vi "Check_Execution_Row.vi"(0 "Execution Row":T1 {"Carrier_2 Q (l/min)" format="%#.2f"; "Row Duration (mins)" format="%#.1f"; "Row No" min=0; "Trace Gas Concentration (%)" min=0.0 format="%#_4f"; "Carrier_1 Q (l/min)" format="%#.2f"; "Tunnel Speed" format="%#.2f"; "Start X" format="%#.2f"; "Start Y" format="%#.2f"; "Start Z" format="%#.2f"; "End X" format="%#.2f"; "End Y" format="%#.2f"; "End Z" format="%#.2f"; "Averaging time (min)" min=0.0 format="%#.2f"}, 1 "Earlier Filenames":path[](array[path]), 3 "Synchronization Start No":i32=1 min=1 max=100, 4 "Row Index":i32, 5 "Max Tunnel Speed":dbl format="%.2f") -> (6 "Edited Row":bool, 7 "Execution Row Out":T1 {"Carrier_2 Q (l/min)" format="%#.2f"; "Row Duration (mins)" format="%#.1f"; "Row No" min=0; "Trace Gas Concentration (%)" min=0.0 format="%#_4f"; "Carrier_1 Q (l/min)" format="%#.2f"; "Tunnel Speed" format="%#.2f"; "Start X" format="%#.2f"; "Start Y" format="%#.2f"; "Start Z" format="%#.2f"; "End X" format="%#.2f"; "End Y" format="%#.2f"; "End Z" format="%#.2f"; "Averaging time (min)" min=0.0 format="%#.2f"}, 9 "Continue?":bool, 10 "Error Comments":string)   [LabVIEW 2016]
uses:
  Traverse_cluster.ctl
  Spacing.ctl
  Controls/Multi_run_mode.ctl
  Controls/User_Specific_mode.ctl
  Controls/Home.ctl
  Controls/Tunnel_Coordinates.ctl
  ADAM Client/Sub VIs/ADAM Controls/Channel_names.ctl
  Globals/Extra_Commands_Global.vi
  Globals/Constants_global.vi
  Globals/Trav_pos_global.vi
panel:
  out "Traverse line Out":T1 {"Carrier_2 Q (l/min)" format="%#.2f"; "Row Duration (mins)" format="%#.1f"; "Row No" min=0; "Trace Gas Concentration (%)" min=0.0 format="%#_4f"; "Carrier_1 Q (l/min)" format="%#.2f"; "Tunnel Speed" format="%#.2f"; "Start X" format="%#.2f"; "Start Y" format="%#.2f"; "Start Z" format="%#.2f"; "End X" format="%#.2f"; "End Y" format="%#.2f"; "End Z" format="%#.2f"; "Averaging time (min)" min=0.0 format="%#.2f"}
  out "Fixed Axis":bool[](array[boolean])
  out "Filenames":string[](array[string])
  out "Current Sync Number":i32
  out "Checks":string[](array[string])
  in  "Edit in Excel":bool
  in  "OK":bool
  # "X           Y            Z"
  # "Start"
  # "End"
  # "X           Y            Z"
  # "Start"
  # "End"
  # "X           Y            Z"
  # "Start"
  # "End"
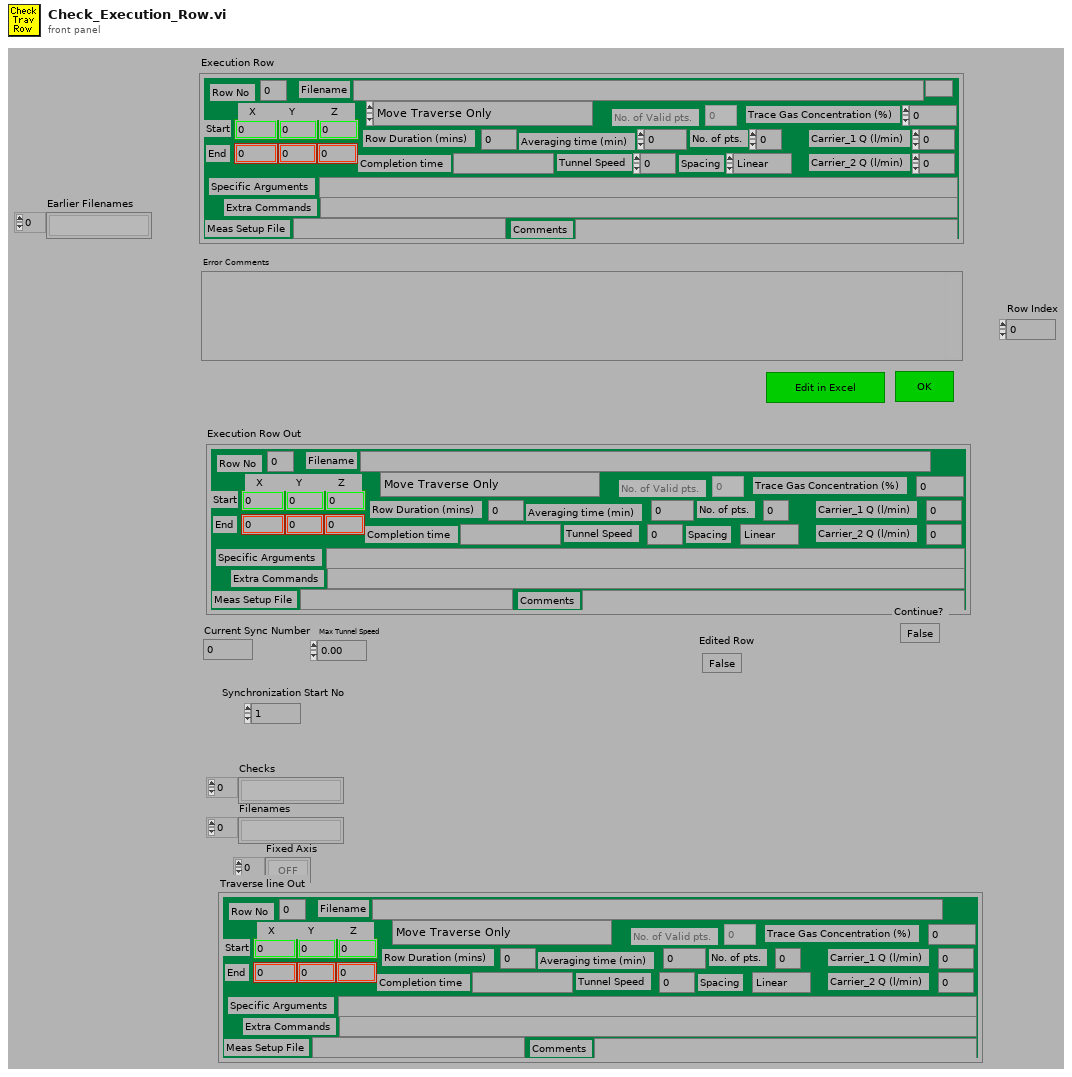
[diagram p1: front panel]
types:
  T1 = typedef "Traverse_cluster.ctl" = cluster{"Start X":sgl, "Start Y":sgl, "Start Z":sgl, "End X":sgl, "End Y":sgl, "End Z":sgl, "No. of pts.":i32, "Spacing":T2, "Filename":path, "Tunnel Speed":dbl, "Averaging time (min)":dbl, "Extra Commands":string, "Carrier_1 Q (l/min)":dbl, "Carrier_2 Q (l/min)":dbl, "Trace Gas Concentration (%)":dbl, "Specific Arguments":string, "Comments":string, "Row No":i32, "Row Type Selector":T3, "Completion time":string, "Row Duration (mins)":dbl, "No. of Valid pts.":i32, "Meas Setup File":string}
  T2 = typedef "Spacing.ctl" = enum16{"Linear", "Log", "Gauss", "Specified", "N/A"}
  T3 = typedef "Multi_run_mode.ctl" = enum16{"Move Traverse Only", "Set Tunnel Speed Only", "Set Source Only", "Set Measurement Conditions", "Single Measurement", "Vertical Profile", "Lateral Profile", "Longitudinal Profile", "Explore Volume", "Multi-Axis Profile", "Auto Calibrate", "Meas Fast FID Bkgnd", "Check Beam Power", "Scanning Valve Measurement", "Run VI Named:", "Set ADAM Ch", "Wait (minutes)", "Send Message", "Synchronize With:", "Fall Back to this Row", "Turn Off Row Repeating", "Blank Row", "Traverse 3D Volume"}
  T4 = enum16{"All Channel Names", "Valid Channel Names"}
  T5 = typedef "User_Specific_mode.ctl" = enum16{"Check VI only", "Run VI"}
  T6 = typedef "Home.ctl" = enum16{"Don't Home", "Home  +X", "Home  -X", "Home  +Y", "Home  -Y", "Home  +Z", "Home  -Z"}
  T7 = typedef "Tunnel_Coordinates.ctl" = enum16{"Work in Tunnel Coordinates", "Work in Model Coordinates"}
  T8 = enum16{"Zero or one", "One", "Zero or more", "One or more"}
  T9 = typedef "Channel_names.ctl" = enum16{"Active Only", "Active + Off", "All Channels"}
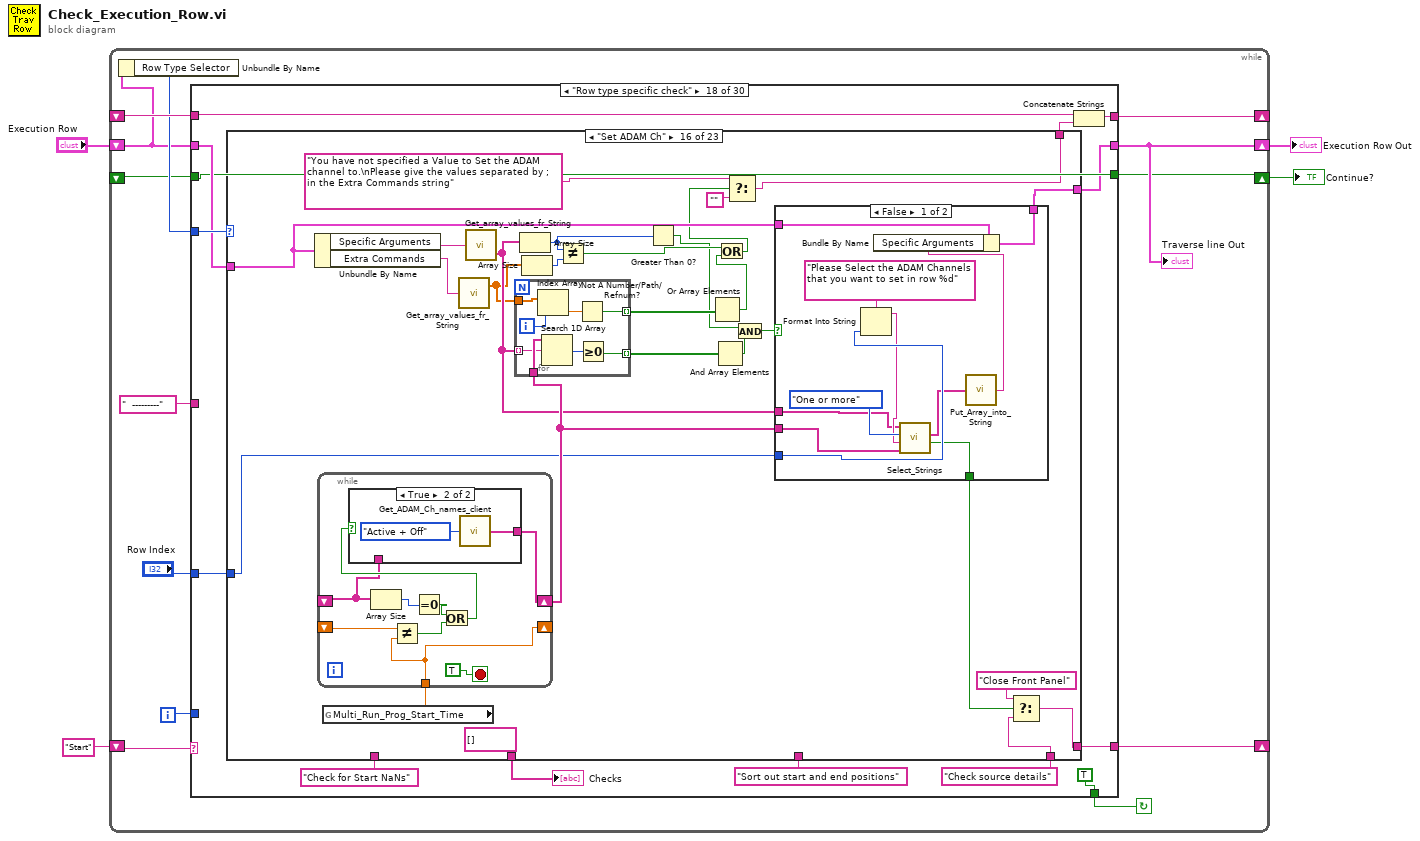
[diagram p0: block diagram]
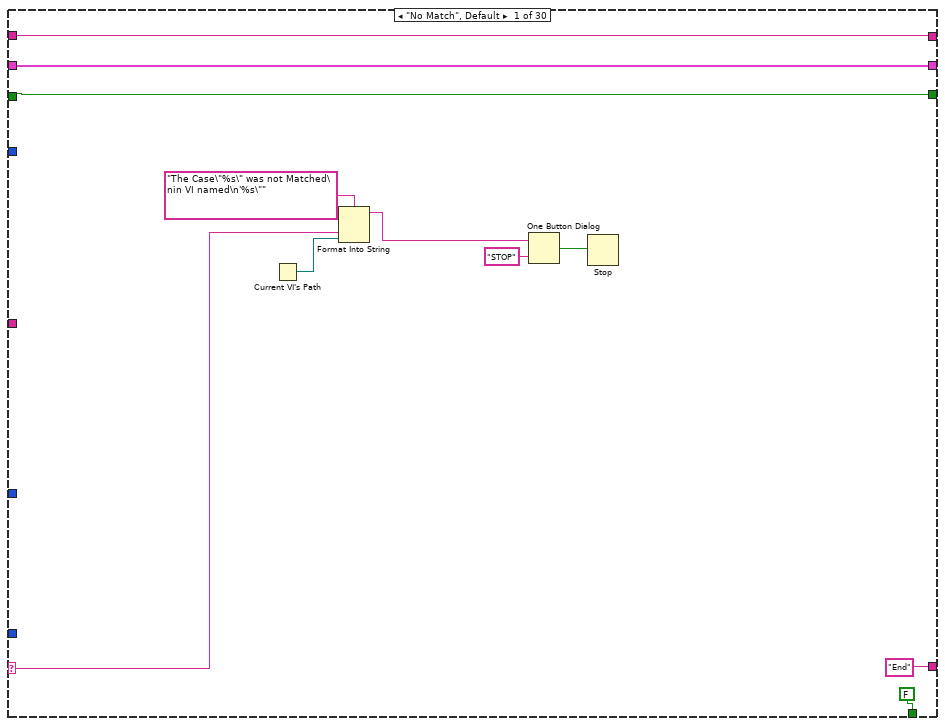
[diagram p2: hidden frame]
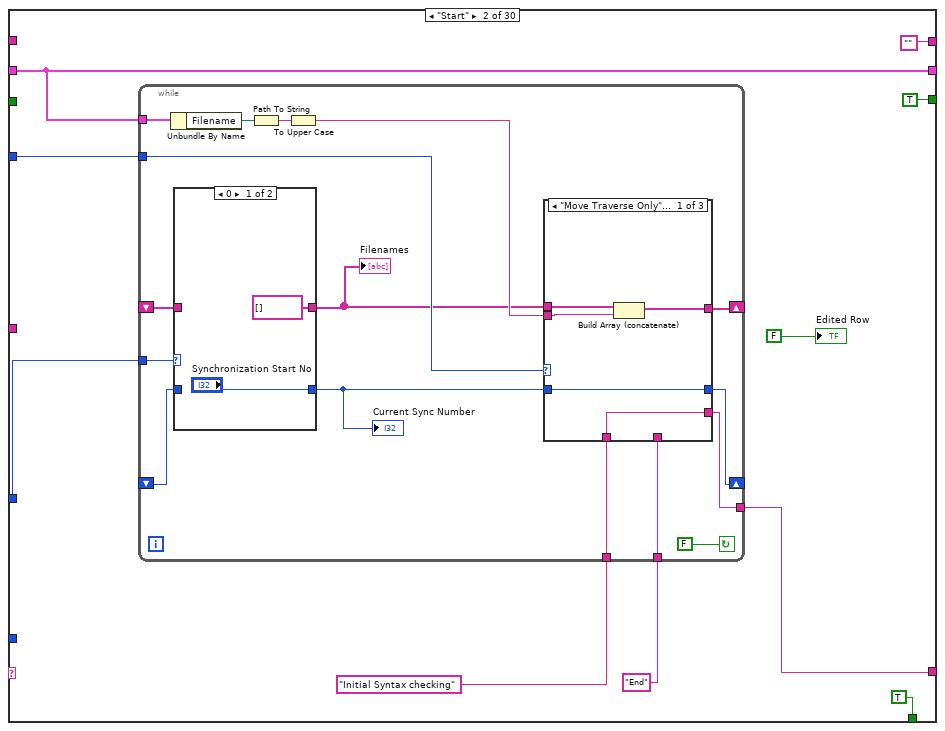
[diagram p3: hidden frame]
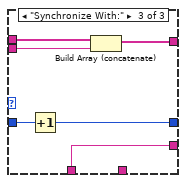
[diagram p6: hidden frame]
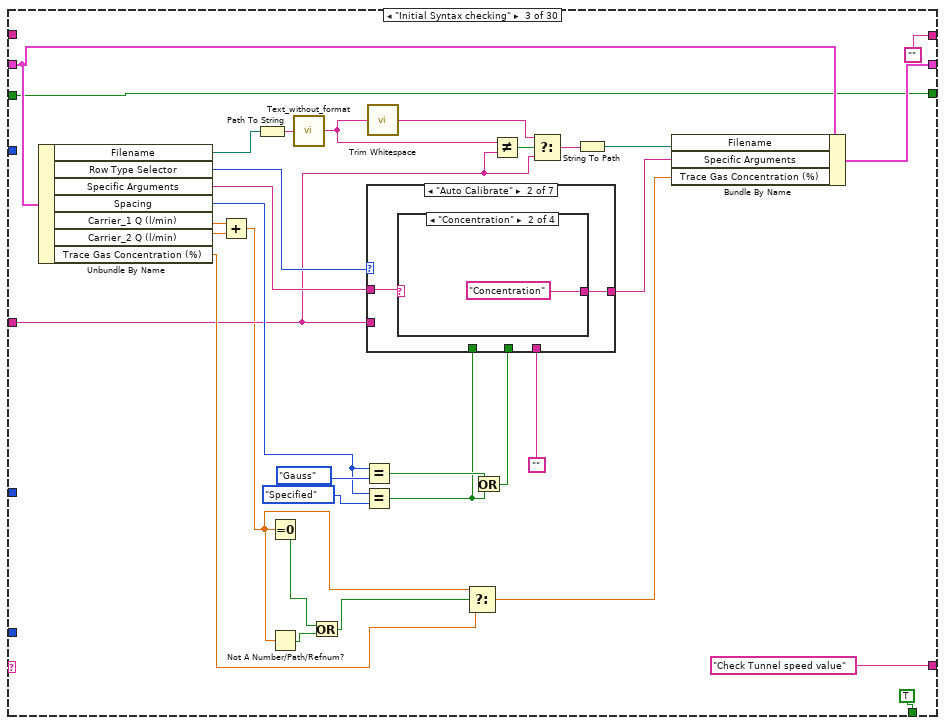
[diagram p7: hidden frame]
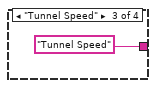
[diagram p10: hidden frame]
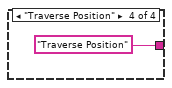
[diagram p11: hidden frame]
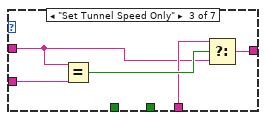
[diagram p12: hidden frame]
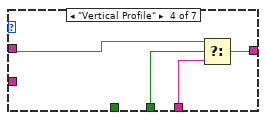
[diagram p13: hidden frame]
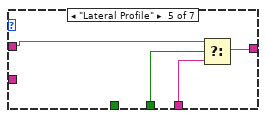
[diagram p14: hidden frame]
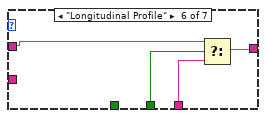
[diagram p15: hidden frame]
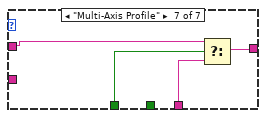
[diagram p16: hidden frame]
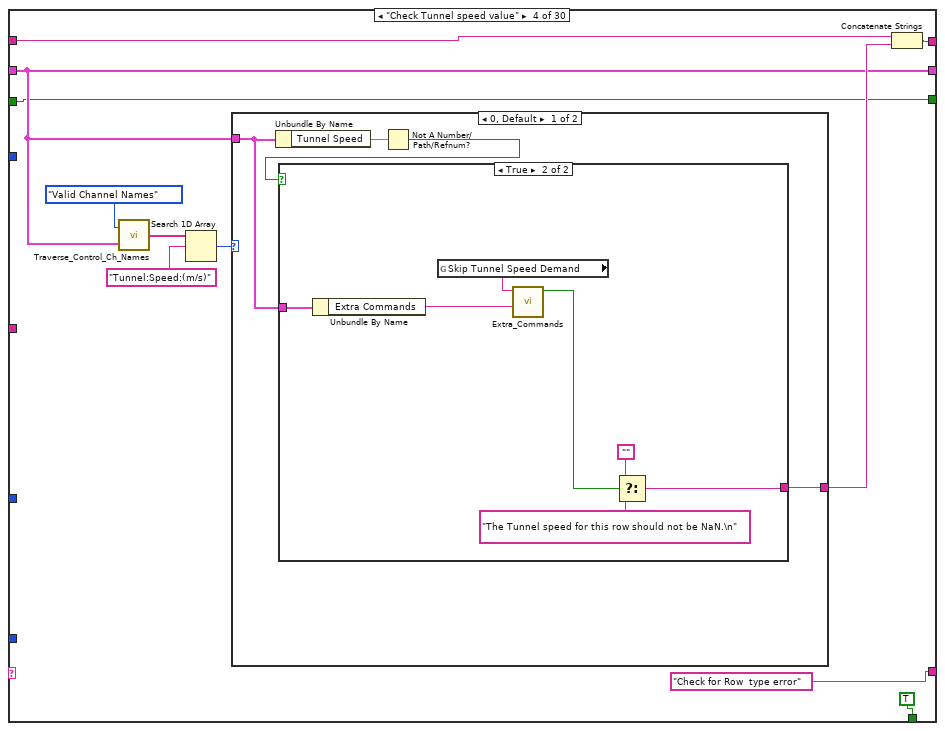
[diagram p17: hidden frame]
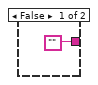
[diagram p18: hidden frame]
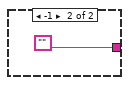
[diagram p19: hidden frame]
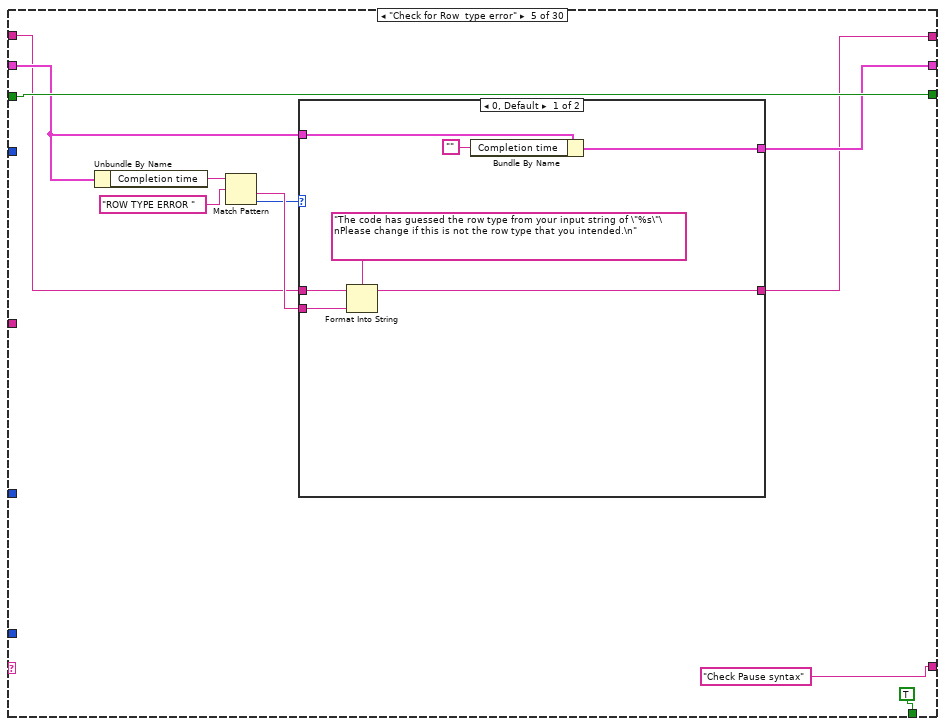
[diagram p20: hidden frame]
diagram:
  n1 = while {
    shift-left: _ -> [w16]
    shift-right: [w17] -> _
    shift-left: "Start" -> [w9]
    shift-right: [w14] -> _
    shift-right: [w8] -> w2
    shift-left: "Execution Row" -> [w5]
    shift-right: [w7] -> w1
    shift-left: _ -> [w6]
    i -> [w10]
    stop <- w15 continue-if-true
    n2 = Unbundle By Name(w5) -> ("Row Type Selector"=w12:T3)
    n3 = case shown="\"Row type specific check\"" w9 {
      tunnel: w5 -> [w23 w32 w99 w136 w160 w192 w217 w264 w294 w324 w357 w433 w460 w499 w555 w587 w595 w634 w1005 w1105 w1142 w1173 w1255 w1266 w1274 w1342 _ w1379 w1386 w1396]
      tunnel: "  ---------" ("f") -> [_ _ w77 _ _ w196 _ _ _ _ _ _ _ _ _ _ _ _ _ _ _ _ _ _ _ _ _ _ _ _]
      tunnel: "Row Index" -> [_ w36 _ _ _ _ w214 _ _ _ _ _ _ _ _ _ _ w628 _ _ _ _ _ _ _ _ _ w1380 _ w1395]
      selector: w9 -> [w18 _ _ _ _ _ _ _ _ _ _ _ _ _ _ _ _ _ _ _ _ _ _ _ _ _ _ _ _ _]
      tunnel: [w22 "" "" w137 w157 w185 w223 w265 w295 w325 w359 w437 w463 w504 w557 w591 w600 w638 w1010 w1115 w1148 w1196 w1254 w1268 w1275 w1348 w1357 w1381 w1391 w1398] -> w17
      tunnel: w12 -> [_ w35 _ _ _ w178 _ _ _ _ _ _ _ _ _ _ w598 w637 w1006 w1103 _ _ _ _ w1279 _ _ _ _ _]
      tunnel: w16 -> [w22 _ _ w138 w158 w187 w224 w266 w296 w326 w360 w438 w464 w505 w557 w590 w601 w639 w1010 w1116 w1149 w1197 w1254 w1269 w1280 w1348 w1357 w1381 w1391 w1398]
      tunnel: [FALSE TRUE TRUE TRUE TRUE TRUE TRUE TRUE TRUE TRUE TRUE TRUE TRUE TRUE TRUE TRUE TRUE TRUE TRUE TRUE TRUE TRUE TRUE TRUE w1271 TRUE TRUE TRUE TRUE FALSE] -> w15
      tunnel: ["End" w33 "Check Tunnel speed value" ("f") "Check for Row  type error" ("f") "Check Pause syntax" ("f") w190 "Check !Use_Axis_Correction" ("f") "Check !Use_2D_Offset_for_Axes" ("f") "Check !Offset Position by dx;dy;dz" ("f") "Check Traverse Setup Name" ("f") "Check Datum Image Extra command" ("f") "Check Trav_Profile_Plug_In" ("f") "Check IF command" ("f") "Check Measurement Setup?" ("f") w559 "Check Maximum tunnel speed" ("f") "Row type specific check" ("f") w635 "Check for position NaNs" ("f") w1106 "Check source details" ("t") "Check source details" ("f") w1251 "check entered filename etc" ("f") w1277 "What to do next?" ("f") w1355 "Initial Syntax checking" "End" "End"] -> w14
      tunnel: w10 -> [_ _ _ _ _ _ _ _ _ _ _ _ _ _ _ _ _ _ _ _ _ _ _ _ _ _ _ _ _ _]
      tunnel: [w23 w32 w80 w136 w161 w180 w216 w264 w294 w324 w357 w433 w460 w499 w555 w586 w595 w629 w1004 w1105 w1142 w1172 w1255 w1266 w1273 w1342 w1350 w1382 w1386 w1394] -> w8
      tunnel: [w19 TRUE w78 w135 w167 w181 w218 w263 w293 w323 w355 w431 w459 w496 w561 w588 w593 w631 w1002 w1104 w1141 w1170 w1256 w1264 w1271 w1341 w1349 w1376 w1385 w1392] -> w7
      tunnel: w6 -> [w19 _ w78 w135 w167 w181 w218 w263 w293 w323 w355 w431 w459 w496 w561 w588 w593 w631 w1002 w1104 w1141 w1170 w1256 w1264 _ w1341 _ w1376 w1385 w1392]
      frame "No Match", Default {
        n4 = Current VI's Path() -> (path=w24:path)
        n5 = Format Into String(format string="The Case\"%s\" was not Matched\nin VI named\n'%s\"" ("Format String"), w18, w24) -> (resulting string=w27:string)  [unwired: 2 in, 1 out]
        n6 = One Button Dialog(message=w27, button name ("OK")="STOP") -> (true=w25:bool)
        n7 = Stop(stop? (T)=w25) -> ()
      }
      frame "Start" {
        n8 = while {
          tunnel: "End" -> [w40]
          tunnel: "Initial Syntax checking" -> [w41]
          tunnel: [w42] -> w33
          tunnel: w32 -> [w49]
          shift-left: _ -> [w48]
          shift-right: [w47] -> _
          tunnel: w35 -> [w53]
          shift-left: _ -> [w52]
          shift-right: [w51] -> _
          tunnel: w36 -> [w54]
          stop <- FALSE continue-if-true
          n9 = Unbundle By Name(w49) -> ("Filename"=w46:path)
          n10 = case shown="0" w54 {
            tunnel: ["Synchronization Start No" w58] -> w50
            tunnel: w52 -> [_ w58]
            tunnel: w48 -> [_ w57]
            tunnel: [string[] [] w57] -> w43
            frame 0 {
            }
            frame 1, Default {
            }
          }
          "Current Sync Number" <- w50
          "Filenames" <- w43
          n11 = Path To String(path=w46) -> (string=w45:string)
          n12 = To Upper Case(1:w45) -> (0:w44:string)
          n13 = case shown="\"Move Traverse Only\", Default" w53 {
            tunnel: w50 -> [w63 w66 w72]
            tunnel: [w63 w66 w71] -> w51
            tunnel: w44 -> [w61 _ w70]
            tunnel: w43 -> [w62 w65 w69]
            tunnel: [w60 w65 w68] -> w47
            tunnel: [w59 w64 w67] -> w42
            tunnel: w41 -> [w59 _ w67]
            tunnel: w40 -> [_ w64 _]
            frame "Move Traverse Only", Default {
              n14 = Build Array (concatenate)(w62, w61) -> (w60:string[])
            }
            frame "Blank Row" {
            }
            frame "Synchronize With:" {
              n15 = Increment(x=w72) -> (x+1=w71:i32)
              n16 = Build Array (concatenate)(w69, w70) -> (w68:string[])
            }
          }
        }
        "Edited Row" <- FALSE ("Editted Row")
      }
      frame "Initial Syntax checking" {
        n17 = Unbundle By Name(w99) -> ("Filename"=w76:path, "Row Type Selector"=w97:T3, "Specific Arguments"=w95:string, "Spacing"=w87:T2, "Carrier_1 Q (l/min)"=w75:dbl, "Carrier_2 Q (l/min)"=w74:dbl, "Trace Gas Concentration (%)"=w93:dbl)
        n18 = Add(x=w75, y=w74) -> (x+y=w73:dbl)
        n19 = Path To String(path=w76) -> (string=w82:string)
        n20 = Equal To 0?(x=w73) -> (x = 0?=w85:bool)
        n21 = Not A Number/Path/Refnum?(number/path/refnum=w73) -> (NaN/Path/Refnum?=w84:bool)
        n22 = call "Text_without_format.vi"("Input string"=w82) -> ("Output string"=w103:string)
        n23 = Or(x=w85, y=w84) -> (x .or. y?=w83:bool)
        n24 = Equal?(x=w87, y=Spacing."Gauss" ("Spacing")) -> (x = y?=w89:bool)
        n25 = Equal?(x=w87, y=Spacing."Specified" ("Spacing")) -> (x = y?=w86:bool)
        n26 = call <vilib>:"Trim Whitespace.vi"("string"=w103) -> ("trimmed string"=w102:string)  [unwired: 1 in]
        n27 = Select(t=w73, s=w83, f=w93) -> (s? t:f=w92:dbl)
        n28 = Or(x=w89, y=w86) -> (x .or. y?=w88:bool)
        n29 = case shown="\"Auto Calibrate\"" w97 {
          tunnel: [w105 w107 w112 w118 w122 w126 w130] -> w96
          tunnel: w95 -> [w105 w106 w113 w120 w124 w128 w132]
          tunnel: "" -> [_ _ w114 w119 w123 w127 w131]
          tunnel: w88 -> [_ _ _ w117 w121 w125 _]
          tunnel: w86 -> [_ _ _ _ _ _ w129]
          tunnel: w77 -> [_ _ w116 _ _ _ _]
          frame "Move Traverse Only", Default {
          }
          frame "Auto Calibrate" {
            n30 = case shown="\"Concentration\"" w106 {
              selector: w106 -> [w108 _ _ _]
              tunnel: [w108 "Concentration" "Tunnel Speed" "Traverse Position"] -> w107
              frame "No Match", Default {
              }
              frame "Concentration" {
              }
              frame "Tunnel Speed" {
              }
              frame "Traverse Position" {
              }
            }
          }
          frame "Set Tunnel Speed Only" {
            n31 = Equal?(x=w113, y=w116) -> (x = y?=w115:bool)
            n32 = Select(t=w114, s=w115, f=w113) -> (s? t:f=w112:string)
          }
          frame "Vertical Profile" {
            n33 = Select(t=w120, s=w117, f=w119) -> (s? t:f=w118:string)
          }
          frame "Lateral Profile" {
            n34 = Select(t=w124, s=w121, f=w123) -> (s? t:f=w122:string)
          }
          frame "Longitudinal Profile" {
            n35 = Select(t=w128, s=w125, f=w127) -> (s? t:f=w126:string)
          }
          frame "Multi-Axis Profile" {
            n36 = Select(t=w132, s=w129, f=w131) -> (s? t:f=w130:string)
          }
        }
        n37 = Not Equal?(x=w103, y=w77) -> (x != y?=w104:bool)
        n38 = Select(t=w102, s=w104, f=w77) -> (s? t:f=w101:string)
        n39 = String To Path(string=w101) -> (path=w81:path)
        n40 = Bundle By Name(cluster=w99, "Filename"=w81, "Specific Arguments"=w96, "Trace Gas Concentration (%)"=w92) -> (w80:T1)
      }
      frame "Check Tunnel speed value" {
        n41 = call "Traverse_Control_Ch_Names.vi"("Traverse line"=w136, "Mode"=T4."Valid Channel Names") -> ("Channel names"=w142:string[])
        n42 = Search 1D Array(1D array=w142, element="Tunnel:Speed:(m/s)" ("Label for value")) -> (index of element=w140:i32)  [unwired: 1 out]
        n43 = case shown="0, Default" w140 {
          tunnel: w136 -> [w145 _]
          tunnel: [w144 ""] -> w139
          frame 0, Default {
            n44 = Unbundle By Name(w145) -> ("Tunnel Speed"=w147:dbl)
            n45 = Not A Number/Path/Refnum?(number/path/refnum=w147) -> (NaN/Path/Refnum?=w146:bool)
            n46 = case shown="True" w146 {
              tunnel: w145 -> [_ w155]
              tunnel: ["" w149] -> w144
              frame False {
              }
              frame True {
                n47 = Unbundle By Name(w155) -> ("Extra Commands"=w153:string)
                n48 = global read "Extra_Commands_Global.vi" "Skip Tunnel Speed Demand"() -> (w154:string)
                n49 = call "Extra_Commands.vi"("String to Search"=w153, "Command"=w154) -> ("Command Found"=w152:bool)  [unwired: 1 in, 4 out]
                n50 = Select(t="", s=w152, f="The Tunnel speed for this row should not be NaN.\n") -> (s? t:f=w149:string)
              }
            }
          }
          frame -1 {
          }
        }
        n51 = Concatenate Strings(w138, w139) -> (w137:string)
      }
      frame "Check for Row  type error" {
        n52 = Unbundle By Name(w160) -> ("Completion time"=w163:string)
        n53 = Match Pattern(string=w163, regular expression="ROW TYPE ERROR " ("format string")) -> (after substring=w162:string, offset past match=w159:i32)  [unwired: 3 out]
        n54 = case shown="0, Default" w159 {
          tunnel: w162 -> [w174 _]
          tunnel: [w172 w176] -> w161
          tunnel: w160 -> [w171 w176]
          tunnel: [w169 w175] -> w157
          tunnel: w158 -> [w168 w175]
          frame 0, Default {
            n55 = Format Into String(format string="The code has guessed the row type from your input string of \"%s\"\nPlease change if this is not the row type that you intended.\n", initial string=w168, w174) -> (resulting string=w169:string)  [unwired: 1 in, 1 out]
            n56 = Bundle By Name(cluster=w171, "Completion time"="") -> (w172:T1)
          }
          frame -1 {
          }
        }
      }
      frame "Check Pause syntax" {
        n57 = Unbundle By Name(w192) -> ("Extra Commands"=w197:string)
        n58 = Equal?(x=Multi_run_mode."Set ADAM Ch" ("Row Type Selector"), y=w178) -> (x = y?=w177:bool)
        n59 = Not Equal?(x=w197, y=w196) -> (x != y?=w198:bool)
        n60 = Select(t=w197, s=w198, f="") -> (s? t:f=w194:string)
        n61 = call <vilib>:"Trim Whitespace.vi"("string"=w194) -> ("trimmed string"=w189:string)  [unwired: 1 in]
        n62 = case shown="False" w177 {
          tunnel: [w200 TRUE] -> w191
          tunnel: w189 -> [w199 _]
          frame False {
            n63 = Equal?(x=w199, y="") -> (x = y?=w200:bool)
          }
          frame True {
          }
        }
        n64 = call "Pause_for_server_ch_val.vi"("Extra command string"=w189, "Simulate/Run"=User_Specific_mode."Check VI only") -> ("Extra command string Out"=w188:string, "Error Comments"=w186:string)
        n65 = Bundle By Name(cluster=w192, "Extra Commands"=w188) -> (w180:T1)
        n66 = Concatenate Strings(w187, w186) -> (w185:string)
        n67 = Select(t="Check Measurement Setup?", s=w191, f="Check Extra Commands") -> (s? t:f=w190:string)
      }
      frame "Check Extra Commands" {
        n68 = global read "Extra_Commands_Global.vi" "Home"() -> (w203:string)
        n69 = Unbundle By Name(w217) -> ("Extra Commands"=w209:string)
        n70 = for {
          N: 4 -> [_]
          tunnel: w209 -> [w242]
          shift-right: [w238] -> w204
          shift-left: "" -> [w239]
          i -> [w244]
          n71 = case shown="0, Default" w244 {
            tunnel: [w247 w249 w251 w253] -> w241
            tunnel: ["The Extra Command \"%s\" should have a numeric argument of (Centre; Intensity) eg 0 ; 0.85 for Gaussian spacing or (Offset) eg 300 for Log \n" ("Format String") "The Extra Command \"%s\" should have a numeric argument.\n" ("Format String") "The Extra Command \"%s\" should have a numeric argument.\n" ("Format String") "The Extra Command \"%s\" should have a numeric argument greater than Zero.\n" ("Format String")] -> w236
            frame 0, Default {
              n72 = global read "Extra_Commands_Global.vi" "Point Spacing Parameters"() -> (w247:string)
            }
            frame 1 {
              n73 = global read "Extra_Commands_Global.vi" "Establish Exp Conditions (s)"() -> (w249:string)
            }
            frame 2 {
              n74 = global read "Extra_Commands_Global.vi" "Minutes Before Repeating Row"() -> (w251:string)
            }
            frame 3 {
              n75 = global read "Extra_Commands_Global.vi" "Puff Duration Sec"() -> (w253:string)
            }
          }
          n76 = call "Extra_Commands.vi"("String to Search"=w242, "Command"=w241) -> ("String Value"=w243:string, "Command Found"=w245:bool)  [unwired: 1 in, 3 out]
          n77 = case shown="True" w245 {
            tunnel: w243 -> [_ w262]
            tunnel: w241 -> [_ w260]
            tunnel: [w254 w257] -> w240
            tunnel: "" -> [w254 w256]
            tunnel: w236 -> [_ w255]
            frame False {
            }
            frame True {
              n78 = Decimal String To Number(string=w262) -> (offset past number=w261:i32)  [unwired: 3 out]
              n79 = Equal To 0?(x=w261) -> (x = 0?=w259:bool)
              n80 = Format Into String(format string=w255, w260) -> (resulting string=w258:string)  [unwired: 2 in, 1 out]
              n81 = Select(t=w258, s=w259, f=w256) -> (s? t:f=w257:string)
            }
          }
          n82 = Concatenate Strings(w240, w239) -> (w238:string)
        }
        n83 = call "Extra_Commands.vi"("String to Search"=w209, "Command"=w203) -> ("String Value"=w207:string, "Command Found"=w208:bool)  [unwired: 1 in, 3 out]
        n84 = case shown="True" w208 {
          tunnel: w207 -> [_ w235]
          tunnel: [TRUE w232] -> w206
          frame False {
          }
          frame True {
            n85 = call "Home_String_to_Enumerated_Type.vi"("String"=w235) -> ("Home"=w234:T6)
            n86 = Not Equal?(x=w234, y=Home."Don't Home" ("Home")) -> (x != y?=w232:bool)
          }
        }
        n87 = call "Trav_Prog_Extra_Commands.vi"() -> ("Extra Commands Array"=w219:string[])  [unwired: 2 out]
        n88 = call "Valid_Extra_Command.vi"("Extra Commands string"=w209, "Valid Commands Array"=w219) -> ("Output String"=w222:string, "Extra Commands string Out"=w215:string)  [unwired: 3 out]
        n89 = Bundle By Name(cluster=w217, "Extra Commands"=w215) -> (w216:T1)
        n90 = call "Skip_If Sd_Error_Below.vi"("String to Search"=w215, "Simulate/Run"=User_Specific_mode."Check VI only", "Measurement setup Applied?"=FALSE, "Row Number"=w214) -> ("Error String"=w211:string)  [unwired: 1 in, 4 out]
        n91 = case shown="False" w206 {
          tunnel: [w228 w230] -> w205
          tunnel: w204 -> [w227 w230]
          tunnel: w203 -> [w229 _]
          frame False {
            n92 = Format Into String(format string="The Extra Command \"%s\" argument should be either\nHome  +X\nHome  -X\nHome  +Y\nHome  -Y\nHome  +Z\nHome  -Z\n" ("Format String"), initial string=w227, w229) -> (resulting string=w228:string)  [unwired: 1 in, 1 out]
          }
          frame True {
          }
        }
        n93 = Concatenate Strings(w224, w222, w205, w211) -> (w223:string)
      }
      frame "Check !Use_Axis_Correction" {
        n94 = Unbundle By Name(w264) -> ("Extra Commands"=w272:string)
        n95 = global read "Extra_Commands_Global.vi" "!Use_Axis_Correction"() -> (w267:string)
        n96 = call "Extra_Commands.vi"("String to Search"=w272, "Command"=w267) -> ("String Value"=w268:string, "Command Found"=w269:bool)  [unwired: 1 in, 3 out]
        n97 = case shown="False" w269 {
          tunnel: w268 -> [_ w283]
          tunnel: w267 -> [_ w277]
          tunnel: w266 -> [w273 w276]
          tunnel: [w273 w275] -> w265
          frame False {
          }
          frame True {
            n98 = call "Get_array_values_fr_String.vi"("String Value"=w283) -> ("String array"=w282:string[])  [unwired: 1 out]
            n99 = Build Array("X", "Y", "Z") -> (w278:string[])
            n100 = for {
              tunnel: w282 -> [w292] mode=indexing
              tunnel: w278 -> [w291]
              tunnel: [w289] -> w274
              stop <- w289 continue-if-true
              n101 = Search 1D Array(1D array=w291, element=w292) -> (index of element=w290:i32)  [unwired: 1 in]
              n102 = Greater Or Equal To 0?(x=w290) -> (x >= 0?=w289:bool)
            }
            n103 = case shown="False" w274 {
              tunnel: [w286 w288] -> w275
              tunnel: w276 -> [w285 w288]
              tunnel: w277 -> [w287 _]
              frame False {
                n104 = Format Into String(format string="The Extra Command \"%s\" argument is invalid Example\n !Use_Axis_Correction = Y" ("Format String"), initial string=w285, w287) -> (resulting string=w286:string)  [unwired: 1 in, 1 out]
              }
              frame True {
              }
            }
          }
        }
      }
      frame "Check !Use_2D_Offset_for_Axes" {
        n105 = Unbundle By Name(w294) -> ("Extra Commands"=w302:string)
        n106 = global read "Extra_Commands_Global.vi" "!Use_2D_Offset_for_Axes"() -> (w297:string)
        n107 = call "Extra_Commands.vi"("String to Search"=w302, "Command"=w297) -> ("String Value"=w298:string, "Command Found"=w299:bool)  [unwired: 1 in, 3 out]
        n108 = case shown="True" w299 {
          tunnel: w298 -> [_ w313]
          tunnel: w297 -> [_ w307]
          tunnel: w296 -> [w303 w306]
          tunnel: [w303 w305] -> w295
          frame False {
          }
          frame True {
            n109 = call "Get_array_values_fr_String.vi"("String Value"=w313) -> ("String array"=w312:string[])  [unwired: 1 out]
            n110 = Build Array("X", "Y", "Z") -> (w308:string[])
            n111 = for {
              tunnel: w312 -> [w322] mode=indexing
              tunnel: w308 -> [w321]
              tunnel: [w319] -> w304
              stop <- w319 continue-if-true
              n112 = Search 1D Array(1D array=w321, element=w322) -> (index of element=w320:i32)  [unwired: 1 in]
              n113 = Greater Or Equal To 0?(x=w320) -> (x >= 0?=w319:bool)
            }
            n114 = case shown="False" w304 {
              tunnel: [w316 w318] -> w305
              tunnel: w306 -> [w315 w318]
              tunnel: w307 -> [w317 _]
              frame False {
                n115 = Format Into String(format string="The Extra Command \"%s\" argument is invalid Example\n!Use_2D_Offset_for_Axes = Y" ("Format String"), initial string=w315, w317) -> (resulting string=w316:string)  [unwired: 1 in, 1 out]
              }
              frame True {
              }
            }
          }
        }
      }
      frame "Check !Offset Position by dx;dy;dz" {
        n116 = Unbundle By Name(w324) -> ("Extra Commands"=w332:string)
        n117 = global read "Extra_Commands_Global.vi" "!Offset Position by dx;dy;dz"() -> (w327:string)
        n118 = call "Extra_Commands.vi"("String to Search"=w332, "Command"=w327) -> ("String Value"=w328:string, "Command Found"=w329:bool)  [unwired: 1 in, 3 out]
        n119 = case shown="True" w329 {
          tunnel: w328 -> [_ w341]
          tunnel: w327 -> [_ w340]
          tunnel: w326 -> [w333 w339]
          tunnel: [w333 w338] -> w325
          frame False {
          }
          frame True {
            n120 = call "Get_array_values_fr_String.vi"("String Value"=w341) -> ("String array"=w337:string[])  [unwired: 1 out]
            n121 = for {
              N: 3 -> [_]
              tunnel: w337 -> [w348] mode=indexing
              tunnel: [w347] -> w335 mode=indexing
              n122 = Fract/Exp String To Number(string=w348) -> (offset past number=w349:i32)  [unwired: 3 in, 1 out]
              n123 = Greater Than 0?(x=w349) -> (x > 0?=w347:bool)
            }
            n124 = And Array Elements(Boolean array=w335) -> (logical AND=w334:bool)
            n125 = case shown="True" w334 {
              tunnel: [w344 w346] -> w338
              tunnel: w339 -> [w343 w346]
              tunnel: w340 -> [w345 _]
              frame False {
                n126 = Format Into String(format string="The Extra Command \"%s\" argument is invalid Example\n!Offset Position by dx;dy;dz = 0;1;0" ("Format String"), initial string=w343, w345) -> (resulting string=w344:string)  [unwired: 1 in, 1 out]
              }
              frame True {
              }
            }
          }
        }
      }
      frame "Check Traverse Setup Name" {
        n127 = Unbundle By Name(w357) -> ("Extra Commands"=w350:string)
        n128 = global read "Extra_Commands_Global.vi" "!Traverse Setup"() -> (w352:string)
        n129 = call "Extra_Commands.vi"("String to Search"=w350, "Command"=w352) -> ("Command Found"=w351:bool)  [unwired: 1 in, 4 out]
        n130 = case shown="True" w351 {
          tunnel: [w361 w366] -> w356
          tunnel: "" -> [w361 w365]
          tunnel: w350 -> [_ w364]
          frame False {
          }
          frame True {
            n131 = call "Which_Trav_Setup.vi"("Extra Command String"=w364) -> ("Traverse Setups"=w363:string[], "XYZ Offset of 2nd Traverse"=w362:sgl[])  [unwired: 1 in, 1 out]
            n132 = stacked-sequence {
              seq-local: [w371 _] -> [_ w401]
              tunnel: [_ w400] -> w366
              tunnel: w365 -> [w373 _]
              tunnel: w363 -> [w368 w406]
              tunnel: w362 -> [_ w402]
              frame #0 {
                n133 = global read "Constants_global.vi" "Traverse folder"() -> (w376:path)
                n134 = Empty Array?(array=w368) -> (empty?=w370:bool)
                n135 = Select(t=string[] [""], s=w370, f=w368) -> (s? t:f=w367:string[])
                n136 = List Folder(path=w376) -> (folder names=w372:string[])  [unwired: 1 in, 5 out]
                n137 = for {
                  tunnel: w367 -> [w392] mode=indexing
                  tunnel: w372 -> [w394]
                  shift-right: [w390] -> w375
                  shift-left: w373 -> [w391]
                  n138 = Search 1D Array(1D array=w394, element=w392) -> (index of element=w393:i32)  [unwired: 1 out]
                  n139 = case shown="-1" w393 {
                    tunnel: w392 -> [_ w398]
                    tunnel: [w395 w397] -> w390
                    tunnel: w391 -> [w395 w396]
                    frame Default {
                    }
                    frame -1 {
                      n140 = Format Into String(format string="%s is not a valid Travese setup.\n", initial string=w396, w398) -> (resulting string=w397:string)  [unwired: 1 in, 1 out]
                    }
                  }
                }
                n141 = Empty String/Path?(string/path=w375) -> (empty?=w374:bool)
                n142 = case shown="False" w374 {
                  tunnel: w372 -> [w383 _]
                  tunnel: [w382 w389] -> w371
                  tunnel: w375 -> [w380 w389]
                  frame False {
                    w377 = "\r\n"
                    n143 = Concatenate Strings(w380, " Valid option are:" ("format string"), w377) -> (w379:string)
                    n144 = for {
                      shift-right: [w386] -> w382
                      shift-left: w379 -> [w387]
                      tunnel: w383 -> [w388] mode=indexing
                      tunnel: "!Traverse Setup =  " ("Substring") -> [w385]
                      tunnel: w377 -> [w384]
                      n145 = Concatenate Strings(w387, w385, w388, w384) -> (w386:string)
                    }
                  }
                  frame True {
                  }
                }
              }
              frame #1 {
                n146 = Array Size(array=w406) -> (size(s)=w405:i32)
                n147 = Greater?(x=w405, y=1) -> (0:w403:bool)
                n148 = case shown="True" w403 {
                  tunnel: w402 -> [_ w411]
                  tunnel: w401 -> [w407 w409]
                  tunnel: [w407 w408] -> w400
                  frame False {
                  }
                  frame True {
                    n149 = Array Size(array=w411) -> (size(s)=w412:i32)
                    n150 = case shown="1, Default" w412 {
                      tunnel: w411 -> [_ _ _ w422]
                      tunnel: [FALSE TRUE TRUE w420] -> w410
                      frame 0 {
                      }
                      frame 1, Default {
                      }
                      frame 2 {
                      }
                      frame 3 {
                        n151 = for {
                          tunnel: w422 -> [w424] mode=indexing
                          tunnel: [w423] -> w421 mode=indexing
                          n152 = Not A Number/Path/Refnum?(number/path/refnum=w424) -> (NaN/Path/Refnum?=w423:bool)
                        }
                        n153 = Or Array Elements(Boolean array=w421) -> (logical OR=w420:bool)
                      }
                    }
                    n154 = case shown="False" w410 {
                      tunnel: w409 -> [w413 w416]
                      tunnel: [w413 w414] -> w408
                      frame False {
                      }
                      frame True {
                        n155 = Concatenate Strings(w416, "Invalid offset for the 2nd traverse.\nExample\n!Traverse Setup =  1st Trav; 2nd Trav; Xoffset; Yoffset; Zoffset;  " ("string")) -> (w414:string)
                      }
                    }
                  }
                }
              }
            }
          }
        }
        n156 = Concatenate Strings(w360, w356) -> (w359:string)
      }
      frame "Check Datum Image Extra command" {
        n157 = Unbundle By Name(w433) -> ("Extra Commands"=w430:string)
        n158 = global read "Extra_Commands_Global.vi" "Datum Image"() -> (w435:string)
        n159 = call "Extra_Commands.vi"("String to Search"=w430, "Command"=w435) -> ("String Value"=w427:string, "Command Found"=w434:bool)  [unwired: 1 in, 3 out]
        n160 = call "Get_array_values_fr_String.vi"("String Value"=w427) -> ("String array"=w426:string[])  [unwired: 1 out]
        n161 = Index Array(array=w426) -> (element=w425:string)  [unwired: 1 in]
        n162 = case shown="True" w434 {
          tunnel: w425 -> [_ w445]
          tunnel: [w439 w442] -> w432
          tunnel: "" -> [w439 w441]
          frame False {
          }
          frame True {
            n163 = Build Path(base path=path "hello", name or relative path=w445) -> (appended path=w444:path)
            n164 = call "Current_Filepath.vi"("Short_Name"="Cal" ("Data Type"), "Filename in"=w444, "Data Type"="Calibrations") -> ("Filename Out"=w440:path)  [unwired: 1 in, 1 out]
            n165 = call "Does_file_exist_(simple).vi"("Pathname"=w440) -> ("exists?"=w443:bool)
            n166 = case shown="False" w443 {
              tunnel: [w449 w452] -> w442
              tunnel: w441 -> [_ w452]
              tunnel: w440 -> [w451 _]
              frame False {
                n167 = Format Into String(format string="Cannot find Datum Image File\n%s", w451) -> (resulting string=w449:string)  [unwired: 2 in, 1 out]
              }
              frame True {
              }
            }
          }
        }
        n168 = Concatenate Strings(w438, w432) -> (w437:string)
      }
      frame "Check Trav_Profile_Plug_In" {
        n169 = global read "Extra_Commands_Global.vi" "Trav_Profile_Plug_In"() -> (w461:string)
        n170 = Unbundle By Name(w460) -> ("Extra Commands"=w458:string)
        n171 = call "Extra_Commands.vi"("String to Search"=w458, "Command"=w461) -> ("String Value"=w455:string, "Command Found"=w456:bool)  [unwired: 1 in, 3 out]
        n172 = case shown="True" w456 {
          tunnel: w455 -> [_ w475]
          tunnel: [w465 w472] -> w453
          tunnel: "" -> [w465 w471]
          frame False {
          }
          frame True {
            n173 = call "Get_array_values_fr_String.vi"("String Value"=w475) -> ("String array"=w468:string[])  [unwired: 1 out]
            n174 = Index Array(array=w468) -> (element=w467:string)  [unwired: 1 in]
            n175 = call "Plug_in_Directories.vi"() -> ("Trav_Profile_Plug_Ins"=w470:path)  [unwired: 2 in, 4 out]
            n176 = List Folder(path=w470) -> (filenames=w469:string[])  [unwired: 1 in, 5 out]
            n177 = Search 1D Array(1D array=w469, element=w467) -> (index of element=w466:i32)  [unwired: 1 out]
            n178 = case shown="Default" w466 {
              tunnel: w467 -> [_ w479]
              tunnel: [w476 w478] -> w474
              tunnel: w471 -> [w476 w477]
              frame Default {
              }
              frame -1 {
                n179 = Format Into String(format string="%s is not a valid Trav_Profile_Plug_In name.\n", initial string=w477, w479) -> (resulting string=w478:string)  [unwired: 1 in, 1 out]
              }
            }
            n180 = Empty String/Path?(string/path=w474) -> (empty?=w473:bool)
            n181 = case shown="False" w473 {
              tunnel: w469 -> [w487 _]
              tunnel: [w486 w493] -> w472
              tunnel: w474 -> [w484 w493]
              frame False {
                w481 = "\r\n"
                n182 = Concatenate Strings(w484, " Valid option are:" ("format string"), w481) -> (w483:string)
                n183 = for {
                  shift-right: [w490] -> w486
                  shift-left: w483 -> [w491]
                  tunnel: w487 -> [w492] mode=indexing
                  tunnel: "!Trav_Profile_Plug_In =  " ("Substring") -> [w489]
                  tunnel: w481 -> [w488]
                  n184 = Concatenate Strings(w491, w489, w492, w488) -> (w490:string)
                }
              }
              frame True {
              }
            }
          }
        }
        n185 = Concatenate Strings(w464, w453) -> (w463:string)
      }
      frame "Check IF command" {
        n186 = Unbundle By Name(w499) -> ("Extra Commands"=w495:string)
        n187 = global read "Extra_Commands_Global.vi" "If Command"() -> (w502:string)
        n188 = call "Extra_Commands.vi"("String to Search"=w495, "Command"=w502) -> ("String Value"=w500:string, "Command Found"=w501:bool)  [unwired: 1 in, 3 out]
        n189 = case shown="True" w501 {
          tunnel: w500 -> [_ w511]
          tunnel: [w506 w510] -> w497
          tunnel: "" -> [w506 w508]
          frame False {
          }
          frame True {
            n190 = call "Get_array_values_fr_String.vi"("String Value"=w511) -> ("Numeric Array"=w507:dbl[], "String array"=w509:string[])
            n191 = Index Array(array=w509, index=0 ("Index")) -> (element=w512:string)
            n192 = case shown="\"Global Value Between\"" w512 {
              tunnel: w511 -> [w517 _ _ _]
              tunnel: [w516 w542 w543 "The !If  command has not been recognised.\nExtra command Example:\n!IF = Time Between;10:45;and;14:00;Execute Row (or) Skip Row\n\n!IF = ADAM Channel Between;Channel Name; 0.5;1.0\n\n!IF = Global Value Between; 0.5;1.0" ("Error Comments")] -> w510
              tunnel: w509 -> [_ w533 w551 _]
              tunnel: w508 -> [_ w526 w544 _]
              tunnel: w507 -> [_ _ _ _]
              frame "Time Between" {
                n193 = Get Date/Time In Seconds() -> (seconds since 1Jan1904=w514:timestamp)
                n194 = To Double Precision Float(number=w514) -> (double precision float=w515:dbl)
                n195 = call "If_Time_arguments.vi"("seconds since 1Jan1904"=w515, "String Value"=w517) -> ("Error Comments"=w516:string)  [unwired: 2 out]
              }
              frame "ADAM Channel Between" {
                n196 = Index Array(array=w533, index=1 ("Index")) -> (element=w536:string)
                n197 = Index Array(array=w533, index=2 ("Index")) -> (element=w532:string)
                n198 = Index Array(array=w533, index=3 ("Index")) -> (element=w531:string)
                n199 = Build Array(w536) -> (w538:string[])
                n200 = Decimal Digit?(1:w532) -> (0:w529:bool)
                n201 = Decimal Digit?(1:w531) -> (0:w530:bool)
                n202 = call "Get_Current_Scan_client.vi"("ADAM Ch Names"=w538) -> ("Numerical Values"=w540:dbl[])  [unwired: 3 out]
                n203 = And(x=w529, y=w530) -> (x .and. y?=w528:bool)
                n204 = Index Array(array=w540, index=0 ("Index")) -> (element=w541:dbl)
                n205 = Select(t=w526, s=w528, f="you must give two limits\n") -> (s? t:f=w522:string)
                n206 = Not A Number/Path/Refnum?(number/path/refnum=w541) -> (NaN/Path/Refnum?=w525:bool)
                n207 = Select(t="Invalid ADAM Channel Name\n", s=w525, f=w526) -> (s? t:f=w523:string)
                n208 = Concatenate Strings(w523, w522) -> (w520:string)
                n209 = Concatenate Strings(w520, "Extra command Example:\n!IF = ADAM Channel Between;Channel Name; 0.5;1.0") -> (w519:string)
                n210 = Empty String/Path?(string/path=w520) -> (empty?=w521:bool)
                n211 = Select(t=w526, s=w521, f=w519) -> (s? t:f=w542:string)
              }
              frame "Global Value Between" {
                n212 = Index Array(array=w551, index=1 ("Index")) -> (element=w550:string)
                n213 = Index Array(array=w551, index=2 ("Index")) -> (element=w549:string)
                n214 = Decimal Digit?(1:w550) -> (0:w547:bool)
                n215 = Decimal Digit?(1:w549) -> (0:w548:bool)
                n216 = And(x=w547, y=w548) -> (x .and. y?=w546:bool)
                n217 = Select(t=w544, s=w546, f="The Extra command IF statement must have two numerical values for the limits\n\nExtra command Example:\n!IF = Global Value Between; 0.5;1.0") -> (s? t:f=w543:string)
              }
              frame "No Match", Default {
              }
            }
          }
        }
        n218 = Concatenate Strings(w505, w497) -> (w504:string)
      }
      frame "Check Measurement Setup?" {
        n219 = Unbundle By Name(w555) -> ("Row Type Selector"=w560:T3, "Specific Arguments"=w558:string)
        n220 = case shown="\"Lateral Profile\"" w560 {
          tunnel: ["Check Measurement Setup" ("t") "Check Measurement Setup" ("t") "Check Measurement Setup" ("t") "Check Measurement Setup" ("t") "Check Measurement Setup" ("t") "Check Measurement Setup" ("t") "Check Measurement Setup" ("t") "Check Measurement Setup" ("t") "Check Measurement Setup" ("t") "Check Measurement Setup" ("t") w573 w582] -> w559
          tunnel: w558 -> [_ _ _ _ _ _ _ _ _ _ w580 _]
          tunnel: "Check Maximum tunnel speed" ("f") -> [_ _ _ _ _ _ _ _ _ _ w574 w582]
          tunnel: w555 -> [_ _ _ _ _ _ _ _ _ _ w577 _]
          frame "Lateral Profile" {
          }
          frame "Traverse 3D Volume" {
          }
          frame "Longitudinal Profile" {
          }
          frame "Explore Volume" {
          }
          frame "Multi-Axis Profile" {
          }
          frame "Vertical Profile" {
          }
          frame "Single Measurement" {
          }
          frame "Scanning Valve Measurement" {
          }
          frame "Auto Calibrate" {
          }
          frame "Meas Fast FID Bkgnd" {
          }
          frame "Run VI Named:" {
            n221 = Match Pattern(string=w580, regular expression=";") -> (before substring=w579:string)  [unwired: 4 out]
            n222 = call <vilib>:"Trim Whitespace.vi"("string"=w579) -> ("trimmed string"=w578:string)  [unwired: 1 in]
            n223 = call "Run_VI_Named_specific.vi"("Run VI Named String"=w578, "Multi Run Row"=w577) -> ("Check Meas Setup?"=w576:bool)  [unwired: 1 in, 8 out]
            n224 = Select(t="Check Measurement Setup", s=w576, f=w574) -> (s? t:f=w573:string)
          }
          frame "Set Tunnel Speed Only", Default {
          }
        }
      }
      frame "Check Measurement Setup" {
        n225 = Unbundle By Name(w587) -> ("Meas Setup File"=w585:string)
        n226 = call "Check_Measurement_Setups.vi"("Measurement Setup String"=w585) -> ("Measurement Setup String Out"=w584:string, "Error Comments"=w583:string)
        n227 = Bundle By Name(cluster=w587, "Meas Setup File"=w584) -> (w586:T1)
        n228 = Concatenate Strings(w590, w583) -> (w591:string)
      }
      frame "Check Maximum tunnel speed" {
        n229 = case shown="\"Auto Calibrate\"" w598 {
          tunnel: w595 -> [w620 _]
          tunnel: [w611 FALSE] -> w597
          tunnel: [w610 0.0] -> w596
          frame "Auto Calibrate" {
            n230 = Unbundle By Name(w620) -> ("Specific Arguments"=w619:string)
            n231 = call "Get_array_values_fr_String.vi"("String Value"=w619) -> ("Numeric Array"=w613:dbl[], "String array"=w618:string[])
            n232 = Index Array(array=w618, index=0 ("Index")) -> (element=w616:string)
            n233 = Equal?(x=w616, y="Tunnel Speed" ("Output Array")) -> (x = y?=w611:bool)
            n234 = Array Subset(array=w613, index=1 ("Array Index")) -> (w612:dbl[])  [unwired: 1 in]
            n235 = Array Max & Min(array=w612) -> (max value=w610:dbl)  [unwired: 3 out]
          }
          frame "Set Tunnel Speed Only", Default {
          }
        }
        n236 = case shown="False" w597 {
          tunnel: [w608 w609] -> w605
          tunnel: w595 -> [w607 _]
          tunnel: w596 -> [_ w609]
          frame False {
            n237 = Unbundle By Name(w607) -> ("Tunnel Speed"=w608:dbl)
          }
          frame True {
          }
        }
        n238 = Greater?(x=w605, y="Max Tunnel Speed") -> (0:w603:bool)
        n239 = Not A Number/Path/Refnum?(number/path/refnum=w605) -> (NaN/Path/Refnum?=w604:bool)
        n240 = Compound Arithmetic op=AND(invert w604, w603) -> (w602:bool)
        n241 = case shown="True" w602 {
          tunnel: w601 -> [w623 w625]
          tunnel: [w623 w624] -> w600
          tunnel: "Max Tunnel Speed" -> [_ w627]
          frame False {
          }
          frame True {
            n242 = Format Into String(format string="The maximum allowable tunnel speed is %.2f m/s.\n" ("Format String"), initial string=w625, w627) -> (resulting string=w624:string)  [unwired: 1 in, 1 out]
          }
        }
      }
      frame "Row type specific check" {
        n243 = case shown="\"Set ADAM Ch\"" w637 {
          tunnel: w634 -> [w648 w657 w661 w665 w670 w675 w682 w689 w700 w708 w722 w728 w833 w838 w842 w880 w932 w960 w965 w969 w981 w985 w991]
          tunnel: [string[] [] string[] [] string[] [] string[] [] w671 w678 w685 w692 w705 w713 w723 w732 w835 string[] [] w859 string[] [] w927 string[] [] string[] [] string[] [] string[] [] string[] [] string[] []] -> w636
          tunnel: [w642 "" "" "" "" "" "" "" w701 w710 "" w726 w829 "" w854 w876 w943 w962 "" w971 "" "" w993] -> w640
          tunnel: [w651 w658 w662 w666 w669 w676 w683 w690 w699 w709 w721 w730 w823 w839 w853 w883 w928 "check entered filename etc" "check entered filename etc" "check entered filename etc" "check entered filename etc" "check entered filename etc" "check entered filename etc"] -> w635
          tunnel: "Check source details" -> [_ w658 w662 _ _ _ _ _ _ _ w721 _ w823 w839 w853 w882 w929 _ _ _ _ _ _]
          tunnel: "Sort out start and end positions" -> [_ _ _ _ _ w676 w683 w690 _ w709 _ w729 _ _ _ _ _ _ _ _ _ _ _]
          tunnel: "Check for Start NaNs" -> [w651 _ _ w666 w669 _ _ _ w699 _ _ w731 _ _ _ _ _ _ _ _ _ _ _]
          tunnel: [w647 w657 w661 w665 w670 w675 w682 w689 w700 w708 w722 w727 w833 w838 w842 w879 w932 w960 w965 w969 w981 w985 w989] -> w629
          tunnel: w628 -> [_ _ _ _ _ _ _ _ _ _ _ _ _ _ _ w885 _ _ _ _ _ _ _]
          frame "Move Traverse Only" {
            n244 = Unbundle By Name(w648) -> ("Specific Arguments"=w649:string)
            n245 = call <vilib>:"Trim Whitespace.vi"("string"=w649) -> ("trimmed string"=w643:string)  [unwired: 1 in]
            n246 = Equal?(x=w643, y="No Backlash") -> (x = y?=w646:bool)
            n247 = Empty String/Path?(string/path=w643) -> (empty?=w645:bool)
            n248 = Or(x=w645, y=w646) -> (x .or. y?=w644:bool)
            n249 = case shown="False" w644 {
              tunnel: w643 -> [w654 _]
              tunnel: [w653 ""] -> w642
              frame False {
                n250 = Format Into String(format string="\"%s\" is an Incorrect Specific Argument. It should either be left blank or say \"No Backlash\"\n", w654) -> (resulting string=w653:string)  [unwired: 2 in, 1 out]
              }
              frame True {
              }
            }
            n251 = Bundle By Name(cluster=w648, "Specific Arguments"=w643) -> (w647:T1)
          }
          frame "Set Tunnel Speed Only" {
          }
          frame "Set Source Only" {
          }
          frame "Set Measurement Conditions" {
          }
          frame "Single Measurement" {
            n252 = Build Array("Averaging:Time:(mins)" ("Label for value"), "Filename:HD:Users" ("Label for value")) -> (w671:string[])
          }
          frame "Vertical Profile" {
            n253 = Build Array("Number:Of:Points" ("Label for value"), "Averaging:Time:(mins)" ("Label for value"), "Filename:HD:Users" ("Label for value")) -> (w678:string[])
          }
          frame "Lateral Profile" {
            n254 = Build Array("Number:Of:Points" ("Label for value"), "Averaging:Time:(mins)" ("Label for value"), "Filename:HD:Users" ("Label for value")) -> (w685:string[])
          }
          frame "Longitudinal Profile" {
            n255 = Build Array("Number:Of:Points" ("Label for value"), "Averaging:Time:(mins)" ("Label for value"), "Filename:HD:Users" ("Label for value")) -> (w692:string[])
          }
          frame "Explore Volume" {
            n256 = Unbundle By Name(w700) -> ("Specific Arguments"=w698:string)
            n257 = Build Array("Averaging:Time:(mins)" ("Label for value"), "Filename:HD:Users" ("Label for value")) -> (w705:string[])
            n258 = Fract/Exp String To Number(string=w698) -> (number=w697:dbl)  [unwired: 4 out]
            n259 = Greater Than 0?(x=w697) -> (x > 0?=w696:bool)
            n260 = Format Into String(format string="\"%s\" is an Incorrect Specific Argument. Please enter the radius of the volume in mm.\n", w698) -> (resulting string=w702:string)  [unwired: 2 in, 1 out]
            n261 = Select(t="", s=w696, f=w702) -> (s? t:f=w701:string)
          }
          frame "Multi-Axis Profile" {
            n262 = Unbundle By Name(w708) -> ("Spacing"=w711:T2)
            n263 = Build Array("Number:Of:Points" ("Label for value"), "Averaging:Time:(mins)" ("Label for value"), "Filename:HD:Users" ("Label for value")) -> (w713:string[])
            n264 = case shown="\"Gauss\"" w711 {
              tunnel: ["" "You are not allowed to specify gaussian spacing for a Multi-Axis profile.\n" "You are not allowed to specify Log spacing for a Multi-Axis profile.\n" "\"N/A\" is not a valid point spacing.\n"] -> w710
              frame "Linear", Default {
              }
              frame "Gauss" {
              }
              frame "Log" {
              }
              frame "N/A" {
              }
            }
          }
          frame "Traverse 3D Volume" {
            n265 = Build Array("Averaging:Time:(mins)" ("Label for value"), "Filename:HD:Users" ("Label for value")) -> (w723:string[])
          }
          frame "Auto Calibrate" {
            n266 = stacked-sequence {
              seq-local: [w735 _ _ _ _] -> [_ _ _ _ w822]
              seq-local: [w734 _ _ _ _] -> [_ w765 _ w811 _]
              seq-local: [w733 _ _ _ _] -> [_ w764 w774 w813 _]
              seq-local: [_ w763 _ _ _] -> [_ _ _ _ w821]
              seq-local: [_ _ w776 _ _] -> [_ _ _ _ w820]
              seq-local: [_ _ _ w804 _] -> [_ _ _ _ w818]
              tunnel: [w744 _ _ _ _] -> w732
              tunnel: w731 -> [w743 _ _ _ _]
              tunnel: [w742 _ _ _ _] -> w730
              tunnel: w729 -> [w741 _ _ _ _]
              tunnel: w728 -> [w740 _ w775 w806 _]
              tunnel: [_ _ w773 _ _] -> w727
              tunnel: [_ _ _ _ w819] -> w726
              frame #0 {
                n267 = Unbundle By Name(w740) -> ("Specific Arguments"=w737:string)
                n268 = call "Get_array_values_fr_String.vi"("String Value"=w737) -> ("Numeric Array"=w734:dbl[], "String array"=w738:string[])
                n269 = Build Array("Tunnel Speed", "Traverse Position", "Concentration") -> (w747:string[])
                n270 = Index Array(array=w738, index=0 ("Index")) -> (element=w736:string)
                n271 = Build Array("Averaging:Time:(mins)" ("Label for value")) -> (w744:string[])
                n272 = Search 1D Array(1D array=w747, element=w736) -> (index of element=w733:i32)  [unwired: 1 out]
                n273 = case shown="0, Default" w733 {
                  tunnel: [w761 w762] -> w742
                  tunnel: w743 -> [w761 _]
                  tunnel: w741 -> [_ w762]
                  frame 0, Default {
                  }
                  frame 1 {
                  }
                }
                n274 = Greater Or Equal To 0?(x=w733) -> (x >= 0?=w745:bool)
                n275 = case shown="False" w745 {
                  tunnel: w747 -> [w752 _]
                  tunnel: [w751 ""] -> w735
                  frame False {
                    n276 = for {
                      shift-right: [w757] -> w754
                      shift-left: "Incorrect Specific Argument. The options are: " -> [w758]
                      tunnel: w752 -> [w759] mode=indexing
                      w756 = "  " ("Substring")
                      n277 = Concatenate Strings(w758, w756, w759, w756) -> (w757:string)
                    }
                    n278 = Concatenate Strings(w754, "\r\n") -> (w751:string)
                  }
                  frame True {
                  }
                }
              }
              frame #1 {
                n279 = Array Size(array=w765) -> (size(s)=w772:i32)
                n280 = Less?(x=w772, y=3) -> (x < y?=w768:bool)
                n281 = Equal To 0?(x=w764) -> (x = 0?=w769:bool)
                n282 = Compound Arithmetic op=AND(w768, w769) -> (w767:bool)
                n283 = Select(t="You need to enter the desired tunnel speeds in the \"Specfic Arguments\" Box   eg.  Tunnel Speed;1;2;3;4\n", s=w767, f="") -> (s? t:f=w763:string)
              }
              frame #2 {
                n284 = global read "Trav_pos_global.vi" "Work in Tunnel Coordinates?"() -> (w787:T7)
                n285 = Unbundle By Name(w775) -> ("Filename"=w780:path)
                n286 = call "Current_Filepath.vi"("Short_Name"="Cal" ("Data Type"), "Filename in"=w780, "Data Type"="Calibrations") -> ("Filename Out"=w778:path)  [unwired: 1 in, 1 out]
                n287 = Equal?(x=w787, y=Tunnel_Coordinates."Work in Model Coordinates" ("Work in Tunnel Coordinates?")) -> (x = y?=w782:bool)
                n288 = Equal?(x=2, y=w774) -> (x = y?=w784:bool)
                n289 = And(x=w782, y=w784) -> (x .and. y?=w783:bool)
                n290 = case shown="True" w783 {
                  tunnel: [w791 w796] -> w779
                  tunnel: w775 -> [w791 w792]
                  frame False {
                  }
                  frame True {
                    n291 = global read "Extra_Commands_Global.vi" "Work in Tunnel Coordinates"() -> (w794:string)
                    n292 = Unbundle By Name(w792) -> ("Extra Commands"=w793:string)
                    n293 = call "Extra_Commands.vi"("String to Search"=w793, "Command"=w794) -> ("Command Found"=w795:bool)  [unwired: 1 in, 4 out]
                    n294 = case shown="False" w795 {
                      tunnel: [w802 w803] -> w796
                      tunnel: w794 -> [w801 _]
                      tunnel: w793 -> [w800 _]
                      tunnel: w792 -> [w798 w803]
                      frame False {
                        n295 = Concatenate Strings(w801, "  " ("string"), w800) -> (w799:string)
                        n296 = Bundle By Name(cluster=w798, "Extra Commands"=w799) -> (w802:T1)
                      }
                      frame True {
                      }
                    }
                  }
                }
                n297 = call "Does_file_exist_(simple).vi"("Pathname"=w778) -> ("exists?"=w790:bool)
                n298 = Select(t="", s=w790, f="The calibration file cannot be found.\n") -> (s? t:f=w776:string)
                n299 = Bundle By Name(cluster=w779, "Filename"=w778) -> (w773:T1)
              }
              frame #3 {
                n300 = Equal?(x=2, y=w813) -> (x = y?=w808:bool)
                n301 = Array Size(array=w811) -> (size(s)=w805:i32)
                n302 = Greater?(x=w805, y=1) -> (0:w809:bool)
                n303 = And(x=w809, y=w808) -> (x .and. y?=w807:bool)
                n304 = case shown="False" w807 {
                  tunnel: w806 -> [_ w817]
                  tunnel: w805 -> [_ _]
                  tunnel: ["" w815] -> w804
                  frame False {
                  }
                  frame True {
                    n305 = Unbundle By Name(w817) -> ("Specific Arguments"=w816:string)
                    n306 = call "Read_FFID_Auto_Calib_Setup.vi"("Specific Argument"=w816) -> ("Error String"=w815:string)  [unwired: 4 out]
                  }
                }
              }
              frame #4 {
                n307 = Concatenate Strings(w822, w821, w820, w818) -> (w819:string)
              }
            }
          }
          frame "Meas Fast FID Bkgnd" {
            n308 = Unbundle By Name(w833) -> ("Specific Arguments"=w828:string)
            n309 = call "Get_array_values_fr_String.vi"("String Value"=w828) -> ("String array"=w827:string[])  [unwired: 1 out]
            n310 = Index Array(array=w827, index=0) -> (element=w825:string)
            n311 = Empty String/Path?(string/path=w825) -> (empty?=w831:bool)
            n312 = Build Array("Averaging:Time:(mins)" ("Label for value")) -> (w835:string[])
            n313 = Equal?(x=w825, y="Use Source Divertor Valve") -> (x = y?=w824:bool)
            n314 = Or(x=w831, y=w824) -> (x .or. y?=w830:bool)
            n315 = case shown="False" w830 {
              tunnel: ["Specific Argument should either be blank or\nUse Source Divertor Valve ; (wait time in seconds optional)" ""] -> w829
              frame False {
              }
              frame True {
              }
            }
          }
          frame "Check Beam Power" {
          }
          frame "Scanning Valve Measurement" {
            w855 = ext -0.5  # lo
            w856 = ext 47.5  # hi
            n316 = Unbundle By Name(w842) -> ("Specific Arguments"=w852:string)
            n317 = call "Get_array_values_fr_String.vi"("String Value"=w852) -> ("Numeric Array"=w851:dbl[], "String array"=w847:string[])
            n318 = Build Array("Averaging:Time:(mins)" ("Label for value"), "Filename:HD:Users" ("Label for value")) -> (w859:string[])
            n319 = Index Array(array=w847, index=0) -> (element=w846:string)
            n320 = Empty String/Path?(string/path=w846) -> (empty?=w844:bool)
            n321 = Index Array(array=w851, index=0) -> (element=w849:dbl)
            n322 = In Range and Coerce(upper limit=w856, x=w849, lower limit=w855) -> (In Range?=w845:bool)  [unwired: 1 out]
            n323 = Compound Arithmetic op=AND(invert w844, w845) -> (w843:bool)
            n324 = Select(t="", s=w843, f="Enter the scanning valve port number between 0 and 47 in the specific arguments box.\n") -> (s? t:f=w854:string)
          }
          frame "Set ADAM Ch" {
            n325 = Unbundle By Name(w880) -> ("Specific Arguments"=w887:string, "Extra Commands"=w875:string)
            n326 = global read "Trav_pos_global.vi" "Multi_Run_Prog_Start_Time"() -> (w862:dbl)
            n327 = while {
              shift-right: [w921] -> w886
              shift-left: _ -> [w917]
              shift-right: [w915] -> _
              shift-left: _ -> [w914]
              tunnel: w862 -> [w915]
              stop <- TRUE stop-if-true
              n328 = Array Size(array=w917) -> (size(s)=w920:i32)
              n329 = Not Equal?(x=w914, y=w915) -> (x != y?=w913:bool)
              n330 = Equal To 0?(x=w920) -> (x = 0?=w919:bool)
              n331 = Or(x=w919, y=w913) -> (x .or. y?=w918:bool)
              n332 = case shown="True" w918 {
                tunnel: [w922 w923] -> w921
                tunnel: w917 -> [w922 _]
                frame False {
                }
                frame True {
                  n333 = call "Get_ADAM_Ch_names_client.vi"("Channel names set"=Channel_names."Active + Off") -> ("Ch names"=w923:string[])
                }
              }
            }
            n334 = call "Get_array_values_fr_String.vi"("String Value"=w875) -> ("Numeric Array"=w871:dbl[])  [unwired: 1 out]
            n335 = call "Get_array_values_fr_String.vi"("String Value"=w887) -> ("String array"=w872:string[])  [unwired: 1 out]
            n336 = for {
              tunnel: w886 -> [w895]
              tunnel: w872 -> [w894] mode=indexing
              tunnel: w871 -> [w890]
              tunnel: [w892] -> w874 mode=indexing
              tunnel: [w891] -> w873 mode=indexing
              i -> [w889]
              n337 = Index Array(array=w890, index=w889) -> (element=w893:dbl)
              n338 = Search 1D Array(1D array=w895, element=w894) -> (index of element=w896:i32)  [unwired: 1 out]
              n339 = Not A Number/Path/Refnum?(number/path/refnum=w893) -> (NaN/Path/Refnum?=w891:bool)
              n340 = Greater Or Equal To 0?(x=w896) -> (x >= 0?=w892:bool)
            }
            n341 = Array Size(array=w872) -> (size(s)=w866:i32)
            n342 = Array Size(array=w871) -> (size(s)=w870:i32)
            n343 = Not Equal?(x=w866, y=w870) -> (x != y?=w868:bool)
            n344 = Greater Than 0?(x=w866) -> (x > 0?=w864:bool)
            n345 = Or Array Elements(Boolean array=w873) -> (logical OR=w869:bool)
            n346 = And Array Elements(Boolean array=w874) -> (logical AND=w865:bool)
            n347 = Or(x=w868, y=w869) -> (x .or. y?=w867:bool)
            n348 = Select(t="You have not specified a Value to Set the ADAM channel to.\nPlease give the values separated by ; in the Extra Commands string", s=w867, f="") -> (s? t:f=w876:string)
            n349 = And(x=w864, y=w865) -> (x .and. y?=w863:bool)
            n350 = case shown="False" w863 {
              tunnel: w886 -> [w907 _]
              tunnel: w872 -> [w899 w909]
              tunnel: w885 -> [w905 _]
              tunnel: [w903 FALSE ("Cancel")] -> w884
              tunnel: w880 -> [w901 w911]
              tunnel: [w900 w910] -> w879
              frame False {
                n351 = Format Into String(format string="Please Select the ADAM Channels that you want to set in row %d", w905) -> (resulting string=w904:string)  [unwired: 2 in, 1 out]
                n352 = call "Select_Strings.vi"("Available Ch names"=w907, "Message"=w904, "Selector mode"=T8."One or more", "Desired Ch names (in)"=w899) -> ("Cancel"=w903:bool, "Selected Channel Names"=w898:string[])  [unwired: 1 in, 2 out]
                n353 = call "Put_Array_into_String.vi"("String array"=w898) -> ("String Value"=w897:string)
                n354 = Bundle By Name(cluster=w901, "Specific Arguments"=w897) -> (w900:T1)
              }
              frame True {
                n355 = call "Put_Array_into_String.vi"("String array"=w909) -> ("String Value"=w908:string)
                n356 = Bundle By Name(cluster=w911, "Specific Arguments"=w908) -> (w910:T1)
              }
            }
            n357 = Select(t="Close Front Panel", s=w884, f=w882) -> (s? t:f=w883:string)
          }
          frame "Run VI Named:" {
            w937 = "Run_VI_Named_specific.vi"
            n358 = Unbundle By Name(w932) -> ("Specific Arguments"=w940:string)
            n359 = global read "Constants_global.vi" "Run VI Folder"() -> (w938:path)
            n360 = Match Pattern(string=w940, regular expression=";") -> (before substring=w941:string)  [unwired: 4 out]
            n361 = call <vilib>:"Trim Whitespace.vi"("string"=w941) -> ("trimmed string"=w933:string)  [unwired: 1 in]
            n362 = call "Run_VI_Named_specific.vi"("Run VI Named String"=w933, "Earlier Filenames"="Earlier Filenames", "Multi Run Row"=w932) -> ("Checks"=w927:string[], "Error String"=w926:string, "Check for start NaNs?"=w931:bool)  [unwired: 6 out]
            n363 = Select(t="Check for Start NaNs" ("Label for value"), s=w931, f=w929) -> (s? t:f=w928:string)
            n364 = Build Path(base path=w938, name or relative path=w933) -> (appended path=w944:path)
            n365 = Not Equal?(x=w933, y=w937) -> (x != y?=w936:bool)
            n366 = call "Does_file_exist_(simple).vi"("Pathname"=w944) -> ("exists?"=w935:bool)
            n367 = And(x=w935, y=w936) -> (x .and. y?=w934:bool)
            n368 = case shown="False" w934 {
              tunnel: [w951 ""] -> w939
              tunnel: w938 -> [w947 _]
              tunnel: w937 -> [w945 _]
              frame False {
                w949 = "\r\n"
                n369 = Build Array(w945) -> (w946:string[])
                n370 = call "List_files_in_order_of_age.vi"("Files to Hide"=w946, "Folder"=w947) -> ("file names"=w948:string[])
                n371 = for {
                  shift-right: [w955] -> w952
                  shift-left: "Cannot find the VI to run. Specific Argument options are:" -> [w956]
                  tunnel: w948 -> [w957] mode=indexing
                  w954 = "  " ("Substring")
                  n372 = Concatenate Strings(w956, w954, w957, w954) -> (w955:string)
                }
                n373 = Concatenate Strings(w952, w949, "Please place one of these strings in the \"Specific Argument\" field.", w949) -> (w951:string)
              }
              frame True {
              }
            }
            n374 = Concatenate Strings(w926, w939) -> (w943:string)
          }
          frame "Wait (minutes)" {
            n375 = Unbundle By Name(w960) -> ("Specific Arguments"=w961:string)
            n376 = call "Wait_Case_Arg.vi"("Specific Argument"=w961) -> ("Error Comments"=w962:string)  [unwired: 1 in, 4 out]
          }
          frame "Send Message" {
          }
          frame "Synchronize With:" {
            n377 = local read "Current Sync Number"() -> (w970:i32)
            n378 = call "Synchronize_Prog_Arg.vi"("Execution Row"=w969) -> ("Error Comments"=w972:string, "Sync No"=w978:i32)  [unwired: 3 out]
            n379 = Format Into String(format string="This should be Synchroisation number %d.\n" ("Format String"), w970) -> (resulting string=w975:string)  [unwired: 2 in, 1 out]
            n380 = Equal?(x=w978, y=w970) -> (x = y?=w977:bool)
            n381 = Select(t="", s=w977, f=w975) -> (s? t:f=w973:string)
            n382 = Concatenate Strings(w973, w972) -> (w971:string)
          }
          frame "Fall Back to this Row" {
          }
          frame "Turn Off Row Repeating" {
          }
          frame "Blank Row" {
            n383 = Unbundle By Name(w991) -> ("Comments"=w997:string)
            n384 = Match Pattern(string=w997, regular expression="(No Match Info)") -> (before substring=w990:string, after substring=w994:string)  [unwired: 3 out]
            n385 = Empty String/Path?(string/path=w994) -> (empty?=w995:bool)
            n386 = Bundle By Name(cluster=w991, "Comments"=w990) -> (w989:T1)
            n387 = Select(t=w994, s=w995, f="The Row Type Selector \"%s\" was not matched. Please select the desired type.\n") -> (s? t:f=w993:string)
          }
        }
        "Checks" <- w636
        n388 = Concatenate Strings(w639, w640) -> (w638:string)
      }
      frame "Sort out start and end positions" {
        n389 = Unbundle By Name(w1005) -> ("Start X"=w1017:sgl, "Start Y"=w1016:sgl, "Start Z"=w1015:sgl, "End X"=w1014:sgl, "End Y"=w1013:sgl, "End Z"=w1012:sgl, "Extra Commands"=w1001:string)
        n390 = call "Which_Trav_Setup.vi"("Extra Command String"=w1001) -> ("Traverse Setups"=w999:string[])  [unwired: 1 in, 2 out]
        n391 = Build Array(w1017, w1016, w1015) -> (w1008:sgl[])
        n392 = Build Array(w1014, w1013, w1012) -> (w1007:sgl[])
        n393 = Index Array(array=w999) -> (element=w1000:string)  [unwired: 1 in]
        n394 = call "Rig_Pict_Display_Pref.vi"("Traverse Name"=w1000) -> ("Which Axis is vertical?"=w1011:enum16{"X Axis", "Y Axis", "Z Axis"})  [unwired: 7 out]
        n395 = case shown="\"Longitudinal Profile\"" w1006 {
          tunnel: [w1057 FALSE w1073 w1086 FALSE] -> w1020
          tunnel: [w1056 FALSE w1072 w1085 FALSE] -> w1019
          tunnel: [w1055 FALSE w1071 w1084 FALSE] -> w1018
          tunnel: w1011 -> [w1054 _ w1070 w1083 _]
          frame "Vertical Profile" {
            n396 = case shown="\"Z Axis\"" w1054 {
              tunnel: [FALSE TRUE TRUE] -> w1057
              tunnel: [TRUE FALSE TRUE] -> w1056
              tunnel: [TRUE TRUE FALSE] -> w1055
              frame "X Axis" {
              }
              frame "Y Axis" {
              }
              frame "Z Axis" {
              }
            }
          }
          frame "Auto Calibrate" {
          }
          frame "Lateral Profile" {
            n397 = case shown="\"Y Axis\"" w1070 {
              tunnel: [TRUE TRUE TRUE] -> w1073
              tunnel: [TRUE TRUE FALSE] -> w1072
              tunnel: [FALSE FALSE TRUE] -> w1071
              frame "X Axis" {
              }
              frame "Y Axis" {
              }
              frame "Z Axis" {
              }
            }
          }
          frame "Longitudinal Profile" {
            n398 = case shown="\"Y Axis\"" w1083 {
              tunnel: [FALSE FALSE FALSE] -> w1086
              tunnel: [TRUE TRUE TRUE] -> w1085
              tunnel: [TRUE TRUE TRUE] -> w1084
              frame "X Axis" {
              }
              frame "Y Axis" {
              }
              frame "Z Axis" {
              }
            }
          }
          frame "Multi-Axis Profile", Default {
          }
        }
        n399 = Build Array(w1020, w1019, w1018) -> (w1009:bool[])
        "Fixed Axis" <- w1009
        n400 = for {
          tunnel: w1009 -> [w1027] mode=indexing
          tunnel: w1008 -> [w1026] mode=indexing
          tunnel: w1007 -> [w1025] mode=indexing
          shift-right: [w1022] -> w1004
          shift-left: w1005 -> [w1023]
          i -> [w1024]
          n401 = case shown="True" w1027 {
            tunnel: w1026 -> [_ w1033]
            tunnel: w1025 -> [_ w1032]
            tunnel: w1024 -> [_ w1031]
            tunnel: w1023 -> [w1028 w1030]
            tunnel: [w1028 w1029] -> w1022
            frame False {
            }
            frame True {
              n402 = Not A Number/Path/Refnum?(number/path/refnum=w1033) -> (NaN/Path/Refnum?=w1034:bool)
              n403 = Not A Number/Path/Refnum?(number/path/refnum=w1032) -> (NaN/Path/Refnum?=w1036:bool)
              n404 = Exclusive Or(1:w1036, 2:w1034) -> (0:w1035:bool)
              n405 = case shown="True" w1035 {
                tunnel: w1034 -> [_ w1044]
                tunnel: w1033 -> [_ w1043]
                tunnel: w1032 -> [_ w1042]
                tunnel: w1031 -> [_ w1041]
                tunnel: w1030 -> [w1037 w1040]
                tunnel: [w1037 w1039] -> w1029
                frame False {
                }
                frame True {
                  n406 = Select(t=w1042, s=w1044, f=w1043) -> (s? t:f=w1038:sgl)
                  n407 = case shown="2" w1041 {
                    tunnel: w1040 -> [w1047 w1050 w1053]
                    tunnel: [w1046 w1049 w1052] -> w1039
                    tunnel: w1038 -> [w1045 w1048 w1051]
                    frame 0, Default {
                      n408 = Bundle By Name(cluster=w1047, "Start X"=w1045, "End X"=w1045) -> (w1046:T1)
                    }
                    frame 1 {
                      n409 = Bundle By Name(cluster=w1050, "Start Y"=w1048, "End Y"=w1048) -> (w1049:T1)
                    }
                    frame 2 {
                      n410 = Bundle By Name(cluster=w1053, "Start Z"=w1051, "End Z"=w1051) -> (w1052:T1)
                    }
                  }
                }
              }
            }
          }
        }
      }
      frame "Check for position NaNs" {
        n411 = global read "Extra_Commands_Global.vi" "Skip Traverse Position Demand"() -> (w1102:string)
        n412 = Unbundle By Name(w1105) -> ("Extra Commands"=w1101:string, "Start X"=w1114:sgl, "Start Y"=w1112:sgl, "Start Z"=w1113:sgl, "End X"=w1111:sgl, "End Y"=w1110:sgl, "End Z"=w1109:sgl)
        n413 = call "Extra_Commands.vi"("String to Search"=w1101, "Command"=w1102) -> ("Command Found"=w1099:bool)  [unwired: 1 in, 4 out]
        n414 = case shown="False" w1099 {
          tunnel: w1114 -> [w1129 _]
          tunnel: w1113 -> [w1128 _]
          tunnel: w1112 -> [w1127 _]
          tunnel: w1111 -> [w1126 _]
          tunnel: w1110 -> [w1125 _]
          tunnel: w1109 -> [w1124 _]
          tunnel: [w1120 w1130] -> w1108
          tunnel: [w1119 TRUE] -> w1107
          tunnel: "" -> [w1118 w1130]
          frame False {
            n415 = Build Array(w1129, w1127, w1128, w1126, w1125, w1124) -> (w1123:sgl[])
            n416 = Not A Number/Path/Refnum?(number/path/refnum=w1123) -> (NaN/Path/Refnum?=w1122:bool[])
            n417 = Or Array Elements(Boolean array=w1122) -> (logical OR=w1119:bool)
            n418 = Select(t="Some of the Start and End positions are NaN.\n" ("f"), s=w1119, f=w1118) -> (s? t:f=w1120:string)
          }
          frame True {
          }
        }
        n419 = case shown="\"Set Tunnel Speed Only\", Default" w1103 {
          tunnel: w1107 -> [_ w1136]
          tunnel: ["Check source details" ("t") w1135] -> w1106
          frame "Multi-Axis Profile" {
          }
          frame "Set Tunnel Speed Only", Default {
            n420 = Select(t="Check source details", s=w1136, f="Check profile rows") -> (s? t:f=w1135:string)
          }
        }
        n421 = Concatenate Strings(w1116, w1108) -> (w1115:string)
      }
      frame "Check for Start NaNs" {
        n422 = Unbundle By Name(w1142) -> ("Extra Commands"=w1138:string, "Start X"=w1147:sgl, "Start Y"=w1145:sgl, "Start Z"=w1146:sgl)
        n423 = global read "Extra_Commands_Global.vi" "Skip Traverse Position Demand"() -> (w1139:string)
        n424 = call "Extra_Commands.vi"("String to Search"=w1138, "Command"=w1139) -> ("Command Found"=w1137:bool)  [unwired: 1 in, 4 out]
        n425 = case shown="False" w1137 {
          tunnel: w1147 -> [w1162 _]
          tunnel: w1146 -> [w1161 _]
          tunnel: w1145 -> [w1160 _]
          tunnel: "" -> [w1158 w1163]
          tunnel: [w1156 w1163] -> w1143
          frame False {
            n426 = Build Array(w1162, w1160, w1161) -> (w1159:sgl[])
            n427 = Not A Number/Path/Refnum?(number/path/refnum=w1159) -> (NaN/Path/Refnum?=w1155:bool[])
            n428 = Boolean To (0,1)(Boolean=w1155) -> (0, 1=w1154:i16[])
            n429 = Add Array Elements(numeric array=w1154) -> (sum=w1153:i16)
            n430 = Greater?(x=w1153, y=i16 2) -> (0:w1151:bool)
            n431 = Select(t="Only up to two of the Start coordinates can be  NaN.\n" ("f"), s=w1151, f=w1158) -> (s? t:f=w1156:string)
          }
          frame True {
          }
        }
        n432 = Concatenate Strings(w1149, w1143) -> (w1148:string)
      }
      frame "Check profile rows" {
        n433 = Unbundle By Name(w1173) -> ("Start X"=w1195:sgl, "Start Y"=w1194:sgl, "Start Z"=w1193:sgl, "End X"=w1192:sgl, "End Y"=w1191:sgl, "End Z"=w1190:sgl, "Specific Arguments"=w1184:string, "Spacing"=w1179:T2, "No. of pts."=w1178:i32)
        n434 = local read "Fixed Axis"() -> (w1177:bool[])
        n435 = Build Array(w1195, w1194, w1193) -> (w1175:sgl[])
        n436 = Build Array(w1192, w1191, w1190) -> (w1176:sgl[])
        n437 = case shown="\"Specified\"" w1179 {
          tunnel: w1184 -> [_ _ _ _ w1230]
          tunnel: ["" w1203 "\"N/A\" is not a valid point spacing.\n" "" w1225] -> w1183
          tunnel: w1178 -> [_ _ _ _ w1229]
          tunnel: w1177 -> [_ w1201 _ _ _]
          tunnel: w1176 -> [_ w1208 _ _ _]
          tunnel: w1175 -> [_ w1207 _ _ _]
          frame "Linear" {
          }
          frame "Log" {
            n438 = for {
              tunnel: w1208 -> [w1212] mode=indexing
              tunnel: w1207 -> [w1211] mode=indexing
              tunnel: [w1210] -> w1206 mode=indexing
              tunnel: w1201 -> [w1209] mode=indexing
              n439 = case shown="False" w1209 {
                tunnel: w1212 -> [w1218 _]
                tunnel: w1211 -> [w1217 _]
                tunnel: [w1213 FALSE] -> w1210
                frame False {
                  w1216 = 0.001 ("y")
                  n440 = Less?(x=w1218, y=w1216) -> (x < y?=w1214:bool)
                  n441 = Less?(x=w1217, y=w1216) -> (x < y?=w1215:bool)
                  n442 = Or(x=w1214, y=w1215) -> (x .or. y?=w1213:bool)
                }
                frame True {
                }
              }
            }
            n443 = Or Array Elements(Boolean array=w1206) -> (logical OR=w1205:bool)
            n444 = Select(t="For log spacing, Start & End positions must be greater than 0.0001.", s=w1205, f="") -> (s? t:f=w1203:string)
          }
          frame "N/A" {
          }
          frame "Gauss" {
          }
          frame "Specified" {
            n445 = call "Get_array_values_fr_String.vi"("String Value"=w1230) -> ("Numeric Array"=w1224:dbl[])  [unwired: 1 out]
            n446 = Array Size(array=w1224) -> (size(s)=w1223:i32)
            n447 = Decrement(x=w1223) -> (x-1=w1222:i32)
            n448 = Equal?(x=w1222, y=w1229) -> (x = y?=w1228:bool)
            n449 = Select(t="", s=w1228, f="The No of points and No of Arguments do not match.\n") -> (s? t:f=w1225:string)
          }
        }
        n450 = for {
          tunnel: w1177 -> [w1236] mode=indexing
          tunnel: w1175 -> [w1235] mode=indexing
          tunnel: w1176 -> [w1234] mode=indexing
          tunnel: [w1233] -> w1189 mode=indexing
          shift-right: [w1231] -> w1168
          shift-left: bool[] [] -> [w1232]
          n451 = case shown="False" w1236 {
            tunnel: w1235 -> [w1240 w1246]
            tunnel: w1234 -> [w1241 w1245]
            tunnel: [TRUE w1244] -> w1233
            tunnel: w1232 -> [w1238 w1243]
            tunnel: [w1237 w1243] -> w1231
            frame False {
              n452 = Not Equal?(x=w1240, y=w1241) -> (x != y?=w1239:bool)
              n453 = Build Array (concatenate)(w1238, w1239) -> (w1237:bool[])
            }
            frame True {
              n454 = Equal?(x=w1246, y=w1245) -> (x = y?=w1244:bool)
            }
          }
        }
        n455 = Array Size(array=w1168) -> (size(s)=w1167:i32)
        n456 = And Array Elements(Boolean array=w1189) -> (logical AND=w1188:bool)
        n457 = Or Array Elements(Boolean array=w1168) -> (logical OR=w1165:bool)
        n458 = Not Equal To 0?(x=w1167) -> (x != 0?=w1166:bool)
        n459 = And(x=w1165, y=w1166) -> (x .and. y?=w1164:bool)
        n460 = call "Create_Pos_array.vi"("Traverse line"=w1173) -> ("Traverse line Out"=w1172:T1, "Error Messages"=w1171:string)  [unwired: 7 out]
        n461 = Select(t="", s=w1188, f="This profile moves more than one axis.\n") -> (s? t:f=w1185:string)
        n462 = Select(t="", s=w1164, f="The start and end points are the same for this profile.\n") -> (s? t:f=w1181:string)
        n463 = Concatenate Strings(w1171, w1181, w1185, w1183) -> (w1198:string)
        n464 = Concatenate Strings(w1197, w1198) -> (w1196:string)
      }
      frame "Check source details" {
        n465 = Unbundle By Name(w1255) -> ("Carrier_1 Q (l/min)"=w1249:dbl, "Carrier_2 Q (l/min)"=w1248:dbl)  [unwired: 1 out]
        n466 = Add(x=w1249, y=w1248) -> (x+y=w1247:dbl)
        n467 = Greater Than 0?(x=w1247) -> (x > 0?=w1253:bool)
        n468 = Select(t="Check source detail 2", s=w1253, f="check entered filename etc") -> (s? t:f=w1251:string)
      }
      frame "Check source detail 2" {
        n469 = Unbundle By Name(w1266) -> ("Trace Gas Concentration (%)"=w1267:dbl)
        n470 = In Range and Coerce(upper limit=ext 2.1099999999999999999 ("hi"), x=w1267, lower limit=ext 0.0 ("lo")) -> (In Range?=w1261:bool)  [unwired: 1 out]
        n471 = Select(t="", s=w1261, f="The Trace Gas Concentration must be within the range of 0 to 2.1%.\n") -> (s? t:f=w1258:string)
        n472 = Concatenate Strings(w1269, w1258) -> (w1268:string)
      }
      frame "check entered filename etc" {
        n473 = local read "Checks"() -> (w1282:string[])
        n474 = for {
          tunnel: w1282 -> [w1289] mode=indexing
          tunnel: [w1294] -> w1283 mode=indexing
          tunnel: w1279 -> [w1293]
          shift-right: [w1291] -> w1273
          shift-left: w1274 -> [w1292]
          tunnel: [w1290] -> w1272 mode=indexing
          n475 = case shown="\"Filename:HD:Users\"" w1289 {
            tunnel: w1292 -> [w1296 w1304 w1328 w1340]
            tunnel: [w1297 w1307 w1334 w1336] -> w1294
            tunnel: w1293 -> [_ _ _ _]
            tunnel: [w1296 w1304 w1326 w1340] -> w1291
            tunnel: [TRUE ("cancelled") TRUE ("cancelled") w1321 TRUE ("cancelled")] -> w1290
            tunnel: w1289 -> [_ _ _ w1338]
            frame "Number:Of:Points" {
              n476 = Unbundle By Name(w1296) -> ("No. of pts."=w1299:i32)
              n477 = Greater?(x=w1299, y=0) -> (0:w1301:bool)
              n478 = Select(t="", s=w1301, f="For a profile the number of points should be more than 0.\n" ("Format String")) -> (s? t:f=w1297:string)
            }
            frame "Averaging:Time:(mins)" {
              n479 = Unbundle By Name(w1304) -> ("Averaging time (min)"=w1306:dbl)
              n480 = Greater Than 0?(x=w1306) -> (x > 0?=w1305:bool)
              n481 = Select(t="", s=w1305, f="The averaging time should be greater than zero.\n" ("Format String")) -> (s? t:f=w1307:string)
            }
            frame "Filename:HD:Users" {
              w1335 = FALSE  # Show Error handler
              n482 = Unbundle By Name(w1328) -> ("Filename"=w1312:path, "Row No"=w1323:i32, "Row Type Selector"=w1319:T3)
              n483 = call "Row_type_selector_string.vi"("Mode"=w1319) -> ("Output string"=w1318:string)
              n484 = call "Current_Filepath.vi"("Short_Name"="Res" ("Data Type"), "Filename in"=w1312, "Data Type"="Results") -> ("Filename Out"=w1313:path)  [unwired: 1 in, 1 out]
              n485 = Path To String(path=w1313) -> (string=w1332:string)
              n486 = Not A Number/Path/Refnum?(number/path/refnum=w1313) -> (NaN/Path/Refnum?=w1316:bool)
              n487 = Match Pattern(string=w1332, regular expression="-------" ("f")) -> (match substring=w1331:string)  [unwired: 4 out]
              n488 = Empty String/Path?(string/path=w1331) -> (empty?=w1317:bool)
              n489 = Format Into String(format string=" For Row  %d %s." ("Comment"), w1323, w1318) -> (resulting string=w1322:string)  [unwired: 2 in, 1 out]
              n490 = Compound Arithmetic op=AND(w1317, invert w1316) -> (w1315:bool)
              n491 = Select(t=w1313, s=w1315, f=path "") -> (s? t:f=w1330:path)
              n492 = call "Results_filename_checker.vi"("Filelength"=45, "Warn if Already Exists"=FALSE, "Comment"=w1322, "Show Error handler"=w1335, "Results file"=w1330) -> ("Error String"=w1334:string, "cancelled"=w1325:bool, "Results file output"=w1327:path)  [unwired: 1 out]
              n493 = Bundle By Name(cluster=w1328, "Filename"=w1327) -> (w1326:T1)
              n494 = Not(x=w1325) -> (.not. x?=w1321:bool)
            }
            frame "No Match", Default {
              n495 = Concatenate Strings(w1338, " Has not been programmed.\n" ("string")) -> (w1336:string)
            }
          }
        }
        n496 = local read "Edited Row"() -> (w1276:bool)
        n497 = And Array Elements(Boolean array=w1272) -> (logical AND=w1271:bool)
        n498 = Concatenate Strings(w1283) -> (w1281:string)
        n499 = Concatenate Strings(w1280, w1281) -> (w1275:string)
        n500 = Empty String/Path?(string/path=w1275) -> (empty?=w1278:bool)
        n501 = case shown="False" w1278 {
          tunnel: ["Open Front Panel" w1287] -> w1277
          tunnel: w1276 -> [_ w1288]
          frame False {
          }
          frame True {
            n502 = Select(t="Close Front Panel", s=w1288, f="End") -> (s? t:f=w1287:string)
          }
        }
      }
      frame "Open Front Panel" {
        w1345 = TRUE  # Front Panel Window:Open
        n503 = Current VI's Path() -> (path=w1346:path)
        n504 = call "Open_Close_Front_Panel.ph.vi"("Front Panel Window:Open"=w1345, "VI path"=w1346) -> ()  [unwired: 2 out]
        n505 = local write "Edited Row"(TRUE ("Editted Row")) -> ()
        n506 = local write "Execution Row"(w1342) -> ()
      }
      frame "What to do next?" {
        w1354 = ""
        w1353 = "[\r\n]"
        n507 = local read "Execution Row"() -> (w1352:T1)
        n508 = Unbundle By Name(w1352) -> ("Row Type Selector"=w1366:T3, "Specific Arguments"=w1361:string, "Extra Commands"=w1359:string)
        n509 = Wait Until Next ms Multiple(millisecond multiple=u32 100) -> ()  [unwired: 1 out]
        n510 = Not Equal?(x=Multi_run_mode."Blank Row" ("Mode"), y=w1366) -> (x != y?=w1362:bool)
        n511 = call "Replace_Character.vi"("Replace with"=w1354, "Input String"=w1361, "Search For"=w1353) -> ("Output string"=w1360:string)  [unwired: 1 out]
        n512 = call "Replace_Character.vi"("Replace with"=w1354, "Input String"=w1359, "Search For"=w1353) -> ("Output string"=w1358:string)  [unwired: 1 out]
        n513 = Compound Arithmetic op=OR("Edit in Excel", "OK") -> (w1363:bool)
        n514 = Bundle By Name(cluster=w1352, "Specific Arguments"=w1360, "Extra Commands"=w1358) -> (w1350:T1)
        n515 = Compound Arithmetic op=AND(w1363, w1362) -> (w1356:bool)
        n516 = Not Equal?(x=w1350, y=w1352) -> (x != y?=w1351:bool)
        n517 = Not(x="Edit in Excel") -> (.not. x?=w1349:bool)
        n518 = case shown="True" w1351 {
          tunnel: w1350 -> [_ w1370]
          frame False {
          }
          frame True {
            n519 = local write "Execution Row"(w1370) -> ()
          }
        }
        n520 = case shown="True" w1349 {
          tunnel: ["Close Front Panel" w1375] -> w1355
          tunnel: w1356 -> [_ w1374]
          frame False {
          }
          frame True {
            n521 = Select(t="Clean Up Row", s=w1374, f="What to do next?") -> (s? t:f=w1375:string)
          }
        }
        "Error Comments" <- w1357
      }
      frame "Clean Up Row" {
        n522 = call "Traverse_Control_Ch_Names.vi"("Mode"=T4."All Channel Names") -> ("Channel names"=w1384:string[])  [unwired: 1 in]
        n523 = call "Trav_Cluster_to_Row.vi"("Traverse line in"=w1379, "Row Number"=w1380, "Channel names"=w1384) -> ("Traverse line Out"=w1382:T1)  [unwired: 4 out]
      }
      frame "Close Front Panel" {
        w1388 = FALSE  # Front Panel Window:Open
        n524 = Current VI's Path() -> (path=w1389:path)
        n525 = call "Open_Close_Front_Panel.ph.vi"("Front Panel Window:Open"=w1388, "VI path"=w1389) -> ()  [unwired: 2 out]
      }
      frame "End" {
        n526 = local read "Edited Row"() -> (w1397:bool)
        n527 = case shown="True" w1397 {
          tunnel: w1396 -> [w1400 w1403]
          tunnel: [w1400 w1402] -> w1394
          tunnel: w1395 -> [_ w1401]
          frame False {
          }
          frame True {
            n528 = call "Traverse_Control_Ch_Names.vi"("Mode"=T4."All Channel Names") -> ("Channel names"=w1404:string[])  [unwired: 1 in]
            n529 = call "Trav_Cluster_to_Row.vi"("Traverse line in"=w1403, "Row Number"=w1401, "Channel names"=w1404) -> ("Traverse line Out"=w1402:T1)  [unwired: 4 out]
          }
        }
        n530 = local write "Error Comments"(w1398) -> ()
      }
    }
    "Traverse line Out" <- w8
  }
  "Execution Row Out" <- w2
  "Continue?" <- w1
